vi "UHR-Fleezers Control (fpga) - 11.4c.vi"() -> ()   [LabVIEW 2012]
doc: "UHR-Fleezers Instrument Control Code (fpga)"
uses:
  <vilib>/Platform/TimedLoop/XDataNode/timing_clust.ctl
  <vilib>/Platform/TimedLoop/XDataNode/nitl_modes.ctl
  <vilib>/Platform/TimedLoop/XDataNode/wakeup.ctl
  <vilib>/rvi/eio/common/nirviEmuTemplateMethod_errors.vi
  <vilib>/rvi/Emulation/niFpgaSctlEmulationGetInTimedLoop.vi
  <vilib>/rvi/DataTransferAndStorage/Container/Common/niFpgaContainerGetUniqueNameForEmu.vi
  <vilib>/rvi/FIFO/Fifo_Resource/nirvififoEmulationSetSize.vi
  <vilib>/rvi/Emulation/niFpgaSctlEmulationFifoFullMgr.vi
  <vilib>/rvi/errors/niFpgaSetErrorForExecOnDevCompSimple.vi
  <vilib>/rvi/eio/common/nirviEmuReportErrorAndStop.vi
  <vilib>/rvi/interface/RandomDataEmulation/nirviRandomDataFPGAFIFO.vi
  <vilib>/rvi/interface/RandomDataEmulation/niFpgaRandomDataHandleErrors.vi
  <vilib>/rvi/Emulation/niFpgaSctlEmulationGlobalWrite.vi
  <vilib>/rvi/Emulation/niFpgaSctlEmulationRegisterWithScheduler.vi
  <vilib>/rvi/Emulation/niFpgaSctlEmulationScheduler.vi
  <vilib>/rvi/Emulation/niFpgaSctlEmulationResourceMgr.vi
  <vilib>/Platform/TimedLoop/XDataNode/XDataNode.xnode
  <vilib>/eio/EIOMethodNode/EIOMethodNode.xnode
  <vilib>/eio/EIONode/EIONode.xnode
  <vilib>/rvi/DataTransferAndStorage/Container/XNode/niFpgaContainer.xnode
  <vilib>/rvi/FIFO/Fifo_Resource/nirvififoEmulationRead.vi
  <vilib>/rvi/interface/RandomDataEmulation/nirviRandomDataFpgaReadWriteTemplate.vi
  <vilib>/rvi/FIFO/Fifo_Resource/nirvififoEmulationWrite.vi
  <vilib>/addons/control/pid/fpga.llb/XNode/niFpgaPID.xnode
  <vilib>/Platform/TimedLoop/XDataNode/XDNodeRunTimeDep.lvlib
panel:
  in  "Tab Control":T1(tab)=enum."Force FB"
  in  "Set 3":bool
  in  "Set 2":bool=TRUE
  in  "Set 1":bool=TRUE
  in  "Trap Pos to FIFO":bool
  in  "N of AI1 Int Acq Sets":i16=2 min=1 max=3 step=1
  out "AI Late Counter":u8
  in  "ai count":u16=400
  in  "+ phase":bool
  in  "Phase count adjustment":i16
  out "Relative phase":i16
  in  "AI to FIFO":bool
  out "BD1 Frequency Out 1":u64
  out "BD1 Frequency Out 2":u64
  out "Trap Pos FIFO Timeout":u16
  out "Trap AI FIFO Timeout":u16
  in  "Trap FIFO Set Timeout":i32
  in  "Tab Control 2":T2(tab)
  in  "RD":bool
  in  "FB1 output high":i16=3000
  in  "FB1 output low":i16
  in  "D1":i16
  in  "I1":i16=5
  in  "P1":i16=10
  in  "Swap F1 and F2":bool
  in  "Cont. Scan":bool
  in  "Abort scan":bool
  in  "Cycles per step":u64
  in  "Scan BD":bool
  in  "Number of scans":u16
  in  "Scan steps":u64
  in  "Scan freq.  increment":i64
  out "Scanning":bool
  in  "Start scan":bool
  in  "OSK Bd 1":bool
  in  "Reset Bd 1":bool
  in  "PMODE":bool
  in  "Direct RF Box \nCommunication":bool
  in  "Data BD 2":u8 format="%08b"
  in  "Data BD 1":u8 format="%08b"
  in  "Address":u8 format="%02x"
  in  "Update Data":bool
  in  "FPGA Controls\n RF Box":bool
  in  "Number Interlace Cycles":u8=2 min=1 max=3
  in  "Interlace Off Parameters":u8=1 min=1 max=3
  in  "Interlace ON/OFF":bool
  out "DIO Relative phase":i16
  in  "Phase count adjustment (DIO)":i16
  in  "+ phase (DIO)":bool
  out "DIO Late Counter":u8
  in  "DIO count 1 (ticks)":u16=400
  in  "DIO count 2 (ticks)":u16=400
  in  "DIO count 3 (ticks)":u16=400
  out "AI2 Y Sum Set 2":i16
  out "AI2 Y Sum Set 1":i16
  in  "FB Setpoint Set 1":i16 min=0 step=1
  in  "FB Reset Set 1":bool
  in  "FB On/Off Set 1":bool
  in  "FB Reset Set 2":bool
  in  "FB On/Off Set 2":bool
  in  "FB Setpoint Set 2":i16 min=0 step=1
  out "Scan I":u64
  in  "Amp switch delay":u8=5
  in  "XY phase ext loop method":bool
  in  "BD 2 Amplitude 1":u16
  in  "BD 1 Amplitude 1":u16
  in  "BD 2 Frequency 1":u64
  in  "BD 1 Frequency 1":u64
  in  "BD 2 Amplitude 2":u16
  in  "BD 1 Amplitude 2":u16
  in  "BD 2 Frequency 2":u64
  in  "BD 1 Frequency 2":u64
  in  "BD 2 Amplitude 3":u16
  in  "BD 1 Amplitude 3":u16
  in  "BD 2 Frequency 3":u64
  in  "BD 1 Frequency 3":u64
  in  "BD 1 Delay (ticks)":u8
  in  "BD 2 Delay (Ticks)":u8 caption="Count(Ticks)"
  in  "Next trap write delay (ticks)":u8 caption="Count(Ticks)"
  in  "Amp switch delay 2":u8=5
  in  "BD 2 Delay (Ticks) 2":u8 caption="Count(Ticks)"
  in  "BD 1 Delay (ticks) 2":u8
  in  "FB2 output high":fxp<+/-,16,1>=0.999969482421875
  in  "FB2 output low":fxp<+/-,16,1>=-1.0
  in  "P2":fxp<+/-,16,8> format="%.11g"
  in  "I2":fxp<+/-,16,8>=10.0 format="%.11g"
  in  "D2":fxp<+/-,16,8> format="%.11g"
  in  "Negate Diff?":bool
  in  "Diff FB Measurement?":bool
  in  "FB Trig Integrate":u32=1
  out "TTrig?":bool
  in  "TTrig Negate Pos":bool=TRUE
  out "Trap Pos FB Int Signal":fxp<+/-,24,9> format="%.18g"
  out "Trap Pos FB Int-Norm Signal":fxp<+/-,16,1> format="%.16g"
  in  "FPGA TTrig Thresh":i64
  in  "FPGA Trap Trig":bool
  out "Trap Pos FB Action":i64
  in  "Trap Pos. FB Offset Factor":i64
  in  "Trap Pos. FB Mult Factor":i64=2
  in  "Trap Pos. FB Reset":bool
  in  "Trap Pos FB Monitor T1 or T2":bool
  in  "AI1 X Scale":u16
  in  "Trap Pos FB Int Count":u16=100
  in  "Trap Pos FB Negate Action":bool
  out "AI1 X Set 2":fxp<+/-,16,1>
  out "AI1 X Set 1":fxp<+/-,16,1>
  in  "Trap Pos. FB SP":fxp<+/-,16,1>
  in  "Force feedback":bool
  out "TTrig Sig":i64
  out "TTrig Fin Thresh":i64
  in  "1D or 2D Scan?":bool
  in  "Abort scan (MCL)":bool
  in  "MCL Scan Axis":bool
  in  "Cont. Scan (MCL)":bool
  out "Scan I (MCL)":u64
  in  "Number of scans (MCL)":u16
  out "Scanning MCL":bool
  in  "Scan steps (MCL)":u64
  in  "Cycles per step (MCL)":u64
  in  "Scan freq.  increment (MCL)":i16
  in  "Start scan (MCL)":bool
  in  "AO2":i16
  in  "AO1":i16
  out "MCL Late Counter":u8
  in  "MCL count":u32=800
  out "MCL Relative Phase":i16
  in  "Phase count adjustment (MCL)":i16
  in  "+ phase (MCL)":bool
  out "APD3 out state":bool
  in  "APD Gate Operating Mode":u8 max=2 step=1
  in  "Invert APD Gate":bool
  in  "APD Gate OFF Count":u16=100
  in  "APD Gate ON Count":u16=300
  out "APD 1 Gate Late Counter":u8
  out "APD 1 Gate Relative Phase":i16
  in  "Phase count adjustment (APD 1 Gate)":i16
  in  "+ phase (APD 1 Gate)":bool
  out "APD 2 Counts 0":u32
  out "APD 2 Counts 1":u32
  out "APD 1 Counts 0":u32
  out "APD 1 Counts 1":u32
  out "APD1 out state":bool
  in  "APD AO scale factor":i16=1
  in  "APD to FIFO":bool
  in  "APD Acq Rate Count":u32=20000000
  out "APD Acq Late Counter":u8
  out "APD Acq Relative Phase":i16
  in  "Phase Count Adjustment (APD Acq)":i16
  in  "+ phase (APD Acq)":bool
  in  "Phase count adjustment (APD 2 Gate)":i16
  out "APD 2 Gate Late Counter":u8
  out "APD 2 Gate Relative Phase":i16
  in  "+ phase (APD 2 Gate)":bool
  out "APD2 out state":bool
  out "APD 3 Counts 0":u32
  out "APD 3 Counts 1":u32
  out "APD 3 Gate Late Counter":u8
  in  "Phase count adjustment (APD 3 Gate)":i16
  out "APD 3 Gate Relative Phase":i16
  in  "+ phase (APD 3 Gate)":bool
  in  "D3":i16
  in  "I3":i16=5
  in  "P3":i16=10
  in  "Green Filter Flipper":bool
  in  "Green FB Count":u16=1200
  out "Green Late Counter":u8
  out "Green FB Relative Phase":i16
  in  "Phase count adjustment (Green FB)":i16=10
  in  "+ phase (Green FB)":bool
  out "Green FB Sum":i16
  in  "Green int current ON count adj":u16=150
  in  "Current Out":u16=30000
  in  "Green FB On/Off":bool
  in  "Green FB Setpoint":i16=250 min=0 step=1
  in  "Green FB Reset":bool
  in  "Operating Mode 2":u8=2 max=2 step=1
  in  "Invert GI 2":bool
  in  "Green interlace OFF count 2":u16=900
  in  "Green interlace ON count 2":u16=300
  out "GI Late Counter 2":u8
  out "GI Relative phase 2":i16
  in  "Phase count adjustment (GI) 2":i16=20
  in  "+ phase (GI) 2":bool
  in  "Green interlace OFF count":u16=100
  out "GI Relative phase":i16
  in  "Phase count adjustment (GI)":i16
  in  "+ phase (GI)":bool
  in  "Green interlace ON count":u16=300
  out "GI Late Counter":u8
  in  "Invert GI":bool
  in  "Operating Mode":u8 max=2 step=1
  in  "+ phase (RI)":bool
  out "RI Relative phase":i16
  out "RI Late Counter":u8
  in  "Red interlace ON count":u16=300
  in  "Red interlace OFF count":u16=100
  in  "Invert RI":bool
  in  "Red Laser Operating Mode":u8 max=2 step=1
  in  "Phase count adjustment (RI)":i16
  out "Red FB Intensity":i16
  in  "RI Current Out":u16=30000
  in  "Red FB On/Off":bool
  in  "D4":i16
  in  "I4":i16=5
  in  "P4":i16=10
  in  "Red FB Setpoint":i16=250 min=0 step=1
  in  "Red FB Reset":bool
  in  "RI Operating Mode 2":u8=2 max=2 step=1
  in  "Invert RI 2":bool
  in  "Phase count adjustment (BI AO)":i16=20
  in  "Blue current ON count adj (AO)":u16=150
  in  "BI Current Out":i16=30000
  in  "Blue FB On/Off":bool
  in  "D5":i16
  in  "I5":i16=5
  in  "P5":i16=10
  in  "Blue FB Setpoint":i16=250 min=0 step=1
  in  "Blue FB Reset":bool
  in  "BI Operating Mode (AO)":u8=2 max=2 step=1
  in  "Invert BI (AO)":bool
  in  "Blue OFF count (AO)":u16=900
  in  "Blue ON count (AO)":u16=300
  out "BI Late Counter (AO)":u8
  out "BI Relative phase (AO)":i16
  in  "+ phase (BI AO)":bool
  in  "Phase count adjustment (BI D)":i16
  in  "Blue Laser Operating Mode (D)":u8 max=2 step=1
  in  "Invert BI (D)":bool
  in  "Blue interlace OFF count (D)":u16=100
  in  "Blue interlace ON count (D)":u16=300
  out "Blue Late Counter (D)":u8
  out "BI Relative phase (D)":i16
  in  "+ phase (BI D)":bool
  out "Blue Intensity":i16
  # "Only one of these can be on\nat a time:"
  # "Raster Scan AOD"
  # "1 (X)"
  # "2 (Y)"
  # "IR Intensity Feedback (RF BD 1)"
  # "FB Gains Set 1"
  # "FB output range 1"
  # "False is usual, True is external loop method"
  # "Parameters if using the external RF switching loop"
  # "Parameters if using the usual internal RF switching method"
  # "FB Triggering Excitation Laser"
  # "Trap Pos. FB Gains"
  # "Trap Pos. FB Range"
  # "AO1 (Y)"
  # "2D"
  # "1D"
  # "AO2 (X)"
  # "APD AO for aligning"
  # "Detection Loop"
  # "Green fluorescent laser digital gate interlacing loop"
  # "0 Forced ON\n1 Forced OFF\n2 Interlacing"
  # "Green FB Gains"
  # "Red fluorescent laser digital gate interlacing loop"
  # "Detection Loop"
  # "0 Forced ON\n1 Forced OFF\n2 Interlacing"
  # "Analog/FB Control Loop\n(Disabled)"
  # "Digital Control Loop"
  # "Blue laser intensity reading"
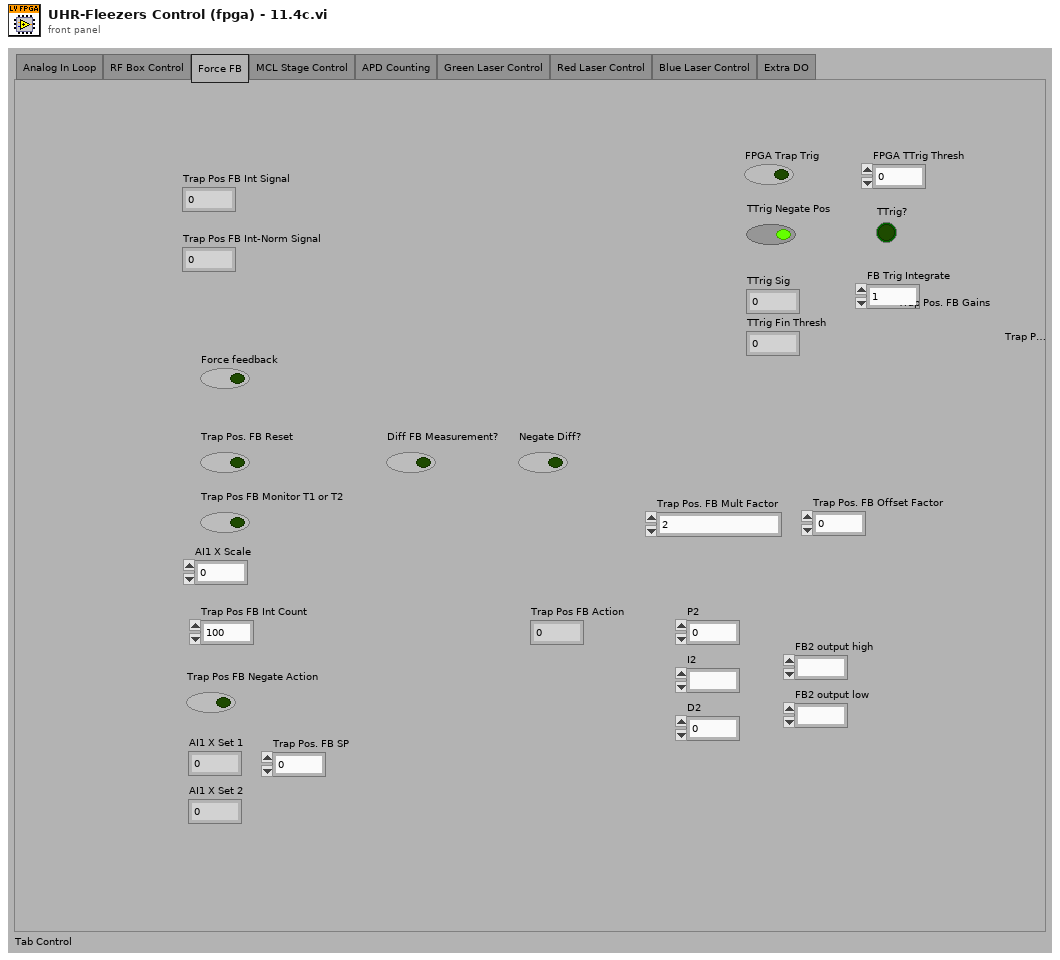
[diagram p1: front panel]
types:
  T1 = enum32{"Analog In Loop", "RF Box Control", "Force FB", "MCL Stage Control", "APD Counting", "Green Laser Control", "Red Laser Control", "Blue Laser Control", "Extra DO"}
  T2 = enum32{"Controls", "Interlacing Frequency and Amplitude Values"}
  T3 = typedef "XDNodeRunTimeDep.lvlib/timing_clust.ctl" = cluster{"Expected End [f-1]":u64, "Actual End [f-1]":u64, "Finished Late? [f-1]":bool, "Expected End [i-1]":u64, "Actual End [i-1]":u64, "Finished Late? [i-1]":bool, "Expected Start [i]":u64, "Actual Start [i]":u64, "Expected Start [f]":u64, "Actual Start [f]":u64, "Source Name":string, "Structure Name":string, "Period":i64, "Deadline":i64, "Offset":i64, "Start":i64, "Priority":i32, "Timeout":i32, "Mode":T4, "Wakeup Reason":T5, "Error":errorcluster, "Source Type":string, "Secondary Source Type":string, "Global End Time":u64, "Global Start Time":u64, "Frame Duration":u64, "Iteration Duration":u64, "Assigned CPU":i32, "I/O Scan Engine Mode":u32}
  T4 = typedef "XDNodeRunTimeDep.lvlib/nitl_modes.ctl" = enum32{"No Change", "Process missed periods, maintain original phase", "Discard missed periods, maintain original phase", "Process missed periods, ignore original phase", "Discard missed periods, ignore original phase"}
  T5 = typedef "XDNodeRunTimeDep.lvlib/wakeup.ctl" = enum32{"Normal", "Aborted", "Asynchronous wakeup", "Timing source error", "Timed loop error", "Timeout"}
  T6 = cluster{"proportional gain (Kc)":i16, "integral gain (Kc*Ts/Ti)":i16, "derivative gain (Kc*Td/Ts)":i16}
  T7 = cluster{"FB1 output high":i16, "FB1 output low":i16}
  T8 = cluster{"P2":fxp<+/-,16,8>, "I2":fxp<+/-,16,8>, "D2":fxp<+/-,16,8>}
  T9 = cluster{"FB2 output high":fxp<+/-,16,1>, "FB2 output low":fxp<+/-,16,1>}
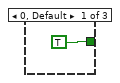
[diagram p3: hidden frame]
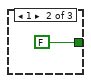
[diagram p4: hidden frame]
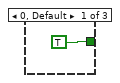
[diagram p5: hidden frame]
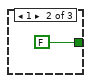
[diagram p6: hidden frame]
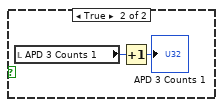
[diagram p7: hidden frame]
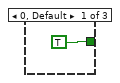
[diagram p8: hidden frame]
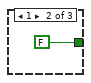
[diagram p9: hidden frame]
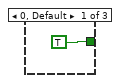
[diagram p10: hidden frame]
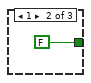
[diagram p11: hidden frame]
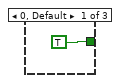
[diagram p12: hidden frame]
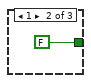
[diagram p13: hidden frame]
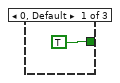
[diagram p14: hidden frame]
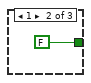
[diagram p15: hidden frame]
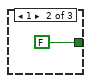
[diagram p18: hidden frame]
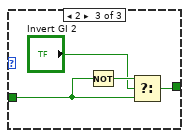
[diagram p19: hidden frame]
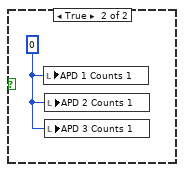
[diagram p20: hidden frame]
diagram:
  w3 = u16 0
  w5 = FALSE
  w2 = FALSE
  # "timing array current index"
  # "timing array"
  # "timing counter (phase adjusted here)"
  # "late counter"
  n1 = while "External XY RF switching timing loop" {
    stop <- FALSE stop-if-true
    # "This loop is stalled until the RF FIFO get a value, which only happens if we are using the external loop RF switching method. With this method we gain additional delay time (because \nwe allow the rest of the main RF loop to procede while this loop waits to send the switch signals - a form of parallelism). Probably this is always the method to use. Helps to simplify \nthe main RF code. If it works reliably, could take out the redundant code in the main RF loop to save space and simplify."
    n2 = xnode "FIFO Read"("Timeout"=-1) -> ("Element"=w15:bool)  [unwired: 1 in, 2 out]
    n3 = flat-sequence "BD 1 (X)" {
      tunnel: w15 -> [w24]
      tunnel: [w24] -> w14
      tunnel: w14 -> [w26]
      tunnel: "Amp switch delay 2" -> [w27]
      frame #0 {
        n4 = call "Wait9"("Count(Ticks)"="BD 1 Delay (ticks) 2") -> ()  [unwired: 1 out]
      }
      frame #1 {
        # "switch frequency"
        n5 = xnode "FPGA I/O Node"("Connector1/DIO36"=w26) -> ()  [unwired: 1 in, 1 out]
      }
      frame #2 {
        # "~5 ticks is usual"
        n6 = call "Wait10"("Count(Ticks)"=w27) -> ()  [unwired: 1 out]
      }
      frame #3 {
        # "this switches amplitude"
        # "switch amplitude"
        # "send udclk high"
        n7 = xnode "FPGA I/O Node"("Connector1/DIO30"=TRUE ("Connector1/DIO15")) -> ()  [unwired: 1 in, 1 out]
      }
      frame #4 {
        # "reset to be ready for next\ncycle"
        # "send udclk low"
        n8 = xnode "FPGA I/O Node"("Connector1/DIO30"=FALSE ("Connector1/DIO15")) -> ()  [unwired: 1 in, 1 out]
      }
    }
    n9 = flat-sequence "BD 2 (Y)" {
      tunnel: w15 -> [w18]
      tunnel: [w18] -> w13
      tunnel: w13 -> [w20]
      tunnel: "Amp switch delay 2" -> [w21]
      frame #0 {
        n10 = call "Wait11"("Count(Ticks)"="BD 2 Delay (Ticks) 2") -> ()  [unwired: 1 out]
      }
      frame #1 {
        # "switch frequency"
        n11 = xnode "FPGA I/O Node"("Connector1/DIO37"=w20) -> ()  [unwired: 1 in, 1 out]
      }
      frame #2 {
        # "~5 ticks is usual"
        n12 = call "Wait12"("Count(Ticks)"=w21) -> ()  [unwired: 1 out]
      }
      frame #3 {
        # "this switches amplitude"
        # "switch amplitude"
        # "send udclk high"
        n13 = xnode "FPGA I/O Node"("Connector1/DIO29"=TRUE ("Connector1/DIO15")) -> ()  [unwired: 1 in, 1 out]
      }
      frame #4 {
        # "reset to be ready for next\ncycle"
        # "send udclk low"
        n14 = xnode "FPGA I/O Node"("Connector1/DIO29"=FALSE ("Connector1/DIO15")) -> ()  [unwired: 1 in, 1 out]
      }
    }
  }
  n15 = flat-sequence "FPGA initialization to do before running any of the loops" {
    tunnel: [u16 0 ("DIO count 3 (ticks)")] -> w1
    tunnel: [w31] -> _
    frame #0 {
      w30 = FALSE ("Enable")
      # "BD 2 (Y)"
      # "BD 1 (X)"
      # "Start up expansion chassis early\nto avoid delays later"
      # "This pin controls udclk on the RF boards.\nWhen initially configuring the boards, this pin needs to be\nconfigured as a high impedance input.  Later it will be switched\nto an output."
      # "Initial setting of DIO data and \naddress to low (before reset).  \nThis needs to happen before the other\ncontrol method loops execute."
      n16 = xnode "FPGA I/O Node"("Chassis2/Mod4/AO0"=u16 0) -> ("Chassis2/Mod1/AI0"=w31:i16)  [unwired: 2 in, 2 out]
      n17 = xnode "FPGA I/O Method Node"("Enable"=w30) -> ()  [unwired: 1 in, 1 out]
      n18 = xnode "FPGA I/O Method Node"("Enable"=w30) -> ()  [unwired: 1 in, 1 out]
      n19 = xnode "FPGA I/O Node"("Connector1/DIO0"=FALSE, "Connector1/DIO1"=FALSE, "Connector1/DIO2"=FALSE, "Connector1/DIO3"=FALSE, "Connector1/DIO4"=FALSE, "Connector1/DIO5"=FALSE, "Connector1/DIO6"=FALSE, "Connector1/DIO7"=FALSE, "Connector1/DIO8"=FALSE, "Connector1/DIO9"=FALSE, "Connector1/DIO10"=FALSE, "Connector1/DIO11"=FALSE, "Connector1/DIO12"=FALSE, "Connector1/DIO13"=FALSE, "Connector1/DIO15"=FALSE, "Connector1/DIO20"=FALSE, "Connector1/DIO21"=FALSE, "Connector1/DIO22"=FALSE, "Connector1/DIO23"=FALSE, "Connector1/DIO24"=FALSE, "Connector1/DIO25"=FALSE, "Connector1/DIO26"=FALSE, "Connector1/DIO27"=FALSE, "Connector1/DIO14"=FALSE) -> ()  [unwired: 24 in, 24 out]
    }
  }
  n20 = local read "AO1"() -> (w10:i16)
  n21 = local read "AO2"() -> (w9:i16)
  n22 = node-c288() -> (w8:T3)  [unwired: 1 in]
  n23 = timed-loop "RF box board DIO control: control bits" {
    timing: w8 -> [_]
    timing-out: [_] -> w7
    tunnel: [w60] -> _
    tunnel: w1 -> [w60]
    stop <- FALSE stop-if-true
    n24 = xnode "FPGA I/O Node"("Connector1/DIO16"="RD", "Connector1/DIO17"="PMODE", "Connector1/DIO18"="OSK Bd 1", "Connector1/DIO19"="Reset Bd 1", "Connector0/DIO3"="Green Filter Flipper") -> ()  [unwired: 5 in, 5 out]
  }
  n25 = while "RF box board DIO control: parallel communication" {
    shift-right: [w73] -> _
    shift-left: w1 -> [w72]
    shift-right: [w71] -> _
    shift-left: FALSE ("Swap F1 and F2") -> [w70]
    stop <- FALSE stop-if-true
    n26 = flat-sequence {
      tunnel: w70 -> [w77]
      tunnel: w72 -> [w75]
      tunnel: [w77] -> w69
      tunnel: [w76] -> w68
      tunnel: [w75] -> w67
      tunnel: [w83] -> w73
      tunnel: [w82] -> w71
      tunnel: w69 -> [w81]
      tunnel: w68 -> [w79]
      tunnel: w67 -> [w78]
      frame #0 {
        n27 = call "Loop Timer"("Count(Ticks)"=w75) -> ("Tick Count(Ticks)"=w76:u16)
      }
      frame #1 {
        n28 = flat-sequence {
          tunnel: ["FPGA Controls\n RF Box"] -> w80
          tunnel: w81 -> [w84]
          tunnel: [w138] -> w83
          tunnel: [w151] -> w82
          tunnel: w80 -> [w150]
          tunnel: w79 -> [w144]
          tunnel: w78 -> [w141]
          frame #0 {
            n29 = case shown="True" "FPGA Controls\n RF Box" {
              tunnel: w84 -> [_ w86]
              frame False {
              }
              frame True {
                n30 = flat-sequence {
                  tunnel: w86 -> [w96]
                  frame #0 {
                    n31 = First Call?() -> (First Call?: T/F=w87:bool)
                    n32 = case shown="True" w87 {
                      frame False {
                      }
                      frame True {
                        # "BD 2"
                        # "BD 1"
                        # "If first time data updated, be sure to set WR high and UDCLK low\nbefore setting data and address bits."
                        n33 = xnode "FPGA I/O Method Node"("Enable"=TRUE) -> ("FPGA I/O Out"=w89:refnum<k21>)  [unwired: 1 in]
                        n34 = xnode "FPGA I/O Method Node"("Enable"=TRUE) -> ("FPGA I/O Out"=w92:refnum<k21>)  [unwired: 1 in]
                        n35 = xnode "FPGA I/O Node"("Connector1/DIO15"=TRUE) -> ()  [unwired: 1 in, 1 out]
                        n36 = xnode "FPGA I/O Node"("I/O Item"=FALSE ("Connector1/DIO30"), "FPGA I/O In"=w89) -> ()  [unwired: 1 out]
                        n37 = xnode "FPGA I/O Node"("I/O Item"=FALSE ("Connector1/DIO30"), "FPGA I/O In"=w92) -> ()  [unwired: 1 out]
                      }
                    }
                  }
                  frame #1 {
                    n38 = case shown="True" "XY phase ext loop method" {
                      tunnel: w96 -> [w98 w110]
                      frame False {
                        # "Usual operation"
                        n39 = flat-sequence "BD 1 (X)" {
                          tunnel: w98 -> [w105]
                          tunnel: "Amp switch delay" -> [w106]
                          frame #0 {
                            n40 = call "Wait6"("Count(Ticks)"="BD 1 Delay (ticks)") -> ()  [unwired: 1 out]
                          }
                          frame #1 {
                            # "switch frequency"
                            n41 = xnode "FPGA I/O Node"("Connector1/DIO36"=w105) -> ()  [unwired: 1 in, 1 out]
                          }
                          frame #2 {
                            # "~5 ticks is usual"
                            n42 = call "Wait4"("Count(Ticks)"=w106) -> ()  [unwired: 1 out]
                          }
                          frame #3 {
                            # "this switches amplitude"
                            # "switch amplitude"
                            # "send udclk high"
                            n43 = xnode "FPGA I/O Node"("Connector1/DIO30"=TRUE ("Connector1/DIO15")) -> ()  [unwired: 1 in, 1 out]
                          }
                          frame #4 {
                            # "reset to be ready for next\ncycle"
                            # "send udclk low"
                            n44 = xnode "FPGA I/O Node"("Connector1/DIO30"=FALSE ("Connector1/DIO15")) -> ()  [unwired: 1 in, 1 out]
                          }
                        }
                        n45 = flat-sequence "BD 2 (Y)" {
                          tunnel: w98 -> [w100]
                          tunnel: "Amp switch delay" -> [w101]
                          frame #0 {
                            n46 = call "Wait7"("Count(Ticks)"="BD 2 Delay (Ticks)") -> ()  [unwired: 1 out]
                          }
                          frame #1 {
                            # "switch frequency"
                            n47 = xnode "FPGA I/O Node"("Connector1/DIO37"=w100) -> ()  [unwired: 1 in, 1 out]
                          }
                          frame #2 {
                            # "~5 ticks is usual"
                            n48 = call "Wait5"("Count(Ticks)"=w101) -> ()  [unwired: 1 out]
                          }
                          frame #3 {
                            # "this switches amplitude"
                            # "switch amplitude"
                            # "send udclk high"
                            n49 = xnode "FPGA I/O Node"("Connector1/DIO29"=TRUE ("Connector1/DIO15")) -> ()  [unwired: 1 in, 1 out]
                          }
                          frame #4 {
                            # "reset to be ready for next\ncycle"
                            # "send udclk low"
                            n50 = xnode "FPGA I/O Node"("Connector1/DIO29"=FALSE ("Connector1/DIO15")) -> ()  [unwired: 1 in, 1 out]
                          }
                        }
                      }
                      frame True {
                        # "Operation when you need a long delay for either X or Y to synchonize AOD light out phase (> ~100 ticks)."
                        # "Trigger the external loop by sending the boolean FSK value through a FIFO"
                        n51 = xnode "FIFO Write"("Element"=w110, "Timeout"=-1) -> ()  [unwired: 1 in, 2 out]
                      }
                    }
                  }
                }
              }
            }
          }
          frame #1 {
            # "This is the prior cycle's on time"
            # "increment timing\nindex, reset to 0 if \nend of matrix"
            # "Reset to begginning (1) when number of cycles reached."
            # "timing index"
            # "build byte stacks for writing data\n(must correspond to addresses array constant)"
            # "Timing housekeeping"
            # "Adjust phase if late\n(maintains constant phase relationship between cycles)"
            n52 = Bundle("FB1 output high"="FB1 output high", "FB1 output low"="FB1 output low") -> (w111:T7)  [unwired: 1 in]
            n53 = Bundle("P1"="P1", "I1"="I1", "D1"="D1") -> (w112:cluster{"P1":i16, "I1":i16, "D1":i16})  [unwired: 1 in]
            n54 = feedback #1(u8 0 ("t")) -> (w147:u8)
            n55 = Increment(x=w147) -> (x+1=w191:u8)
            n56 = Increment(x="Number Interlace Cycles") -> (x+1=w186:u8)
            n57 = Equal?(x=w191, y=w186) -> (x = y?=w193:bool)
            n58 = Select(t=u8 1, s=w193, f=w191) -> (s? t:f=w146:u8)
            n59 = feedback-in #1(w146) -> ()
            n60 = Increment(x=w146) -> (x+1=w188:u8)
            n61 = Equal?(x=w188, y=w186) -> (x = y?=w189:bool)
            n62 = Select(t=u8 1, s=w189, f=w188) -> (s? t:f=w185:u8)
            n63 = Select(t=w185, s="Interlace ON/OFF", f="Interlace Off Parameters") -> (s? t:f=w169:u8)
            n64 = case shown="1, Default" w169 {
              tunnel: [w270 "BD 1 Frequency 2" "BD 1 Frequency 3"] -> w181
              tunnel: [w269 "BD 2 Frequency 2" "BD 2 Frequency 3"] -> w170
              tunnel: ["BD 2 Amplitude 1" "BD 2 Amplitude 2" "BD 2 Amplitude 3"] -> w126
              tunnel: [w258 w429 "BD 1 Amplitude 3"] -> w129
              tunnel: w112 -> [w232 w426 _]
              tunnel: w111 -> [w233 w425 _]
              frame 1, Default {
                w249 = fxp<+/-,24,9> 0.0 ("AI1 X Set 2")
                w242 = u16 0
                w265 = u64 0 ("f")
                # "This signal integration happens no matter what\nso that correct setpoints can be chosen before \nturning on the FB."
                # "Trap 1"
                n65 = local read "AI1 X Set 2"() -> (w245:fxp<+/-,16,1>)
                n66 = local read "AI1 X Set 1"() -> (w246:fxp<+/-,16,1>)
                n67 = local read "Scanning"() -> (w271:bool)
                n68 = Or(x=w271, y="Start scan") -> (x .or. y?=w263:bool)
                n69 = case shown="False" "Diff FB Measurement?" {
                  tunnel: w245 -> [w279 w288]
                  tunnel: w246 -> [w278 w289]
                  tunnel: [w276 w280] -> w247
                  frame False {
                    n70 = Select(t=w278, s="Trap Pos FB Monitor T1 or T2", f=w279) -> (s? t:f=w276:fxp<+/-,16,1>)
                  }
                  frame True {
                    n71 = Subtract(x=w289, y=w288) -> (x-y=w281:fxp<+/-,17,2>)
                    n72 = Not(x="Negate Diff?") -> (.not. x?=w287:bool)
                    n73 = Boolean To (0,1)(Boolean="Negate Diff?") -> (0, 1=w285:i16)
                    n74 = Boolean To (0,1)(Boolean=w287) -> (0, 1=w286:i16)
                    n75 = Negate(x=w285) -> (-x=w284:i16)
                    n76 = Add(x=w284, y=w286) -> (x+y=w282:i16)
                    n77 = Multiply(x=w282, y=w281) -> (x*y=w280:fxp<+/-,32,17>)
                  }
                }
                n78 = Not(x="Abort scan") -> (.not. x?=w261:bool)
                n79 = And(x=w261, y=w263) -> (x .and. y?=w260:bool)
                n80 = case "For raster scanning" shown="True" w260 {
                  tunnel: [u64 0 w415] -> w266
                  tunnel: "Start scan" -> [_ w400]
                  frame False {
                    n81 = local write "Scanning"(FALSE ("scanning")) -> ()
                  }
                  frame True {
                    w384 = i64 0
                    w383 = u64 0
                    # "scan incr."
                    # "freq. incr. mult."
                    # "count steps"
                    # "count number of cycles"
                    n82 = feedback #2(w383) -> (w412:u64)
                    n83 = Select(t=w383, s=w400, f=w412) -> (s? t:f=w414:u64)
                    n84 = Increment(x=w414) -> (x+1=w411:u64)
                    n85 = Greater?(x="Cycles per step", y=w411) -> (0:w393:bool)
                    n86 = Select(t=w411, s=w393, f=w383) -> (s? t:f=w410:u64)
                    n87 = feedback-in #2(w410) -> ()
                    n88 = feedback #3(w383) -> (w409:u64)
                    n89 = Select(t=w383, s=w400, f=w409) -> (s? t:f=w404:u64)
                    n90 = Increment(x=w404) -> (x+1=w408:u64)
                    n91 = Add(x="Scan steps", y="Scan steps") -> (x+y=w407:u64)
                    n92 = Select(t=w404, s=w393, f=w408) -> (s? t:f=w388:u64)
                    n93 = Greater?(x=w407, y=w388) -> (0:w387:bool)
                    n94 = Select(t=w388, s=w387, f=w383) -> (s? t:f=w405:u64)
                    n95 = feedback-in #3(w405) -> ()
                    n96 = Equal?(x="Scan steps", y=w388) -> (x = y?=w392:bool)
                    n97 = Greater?(x="Scan steps", y=w404) -> (0:w403:bool)
                    n98 = feedback #4(w384) -> (w406:i64)
                    n99 = Select(t=w384, s=w400, f=w406) -> (s? t:f=w390:i64)
                    n100 = Increment(x=w390) -> (x+1=w402:i64)
                    n101 = Decrement(x=w390) -> (x-1=w401:i64)
                    n102 = Select(t=w402, s=w403, f=w401) -> (s? t:f=w391:i64)
                    n103 = Select(t=w390, s=w392, f=w391) -> (s? t:f=w389:i64)
                    n104 = Select(t=w390, s=w393, f=w389) -> (s? t:f=w385:i64)
                    n105 = Select(t=w385, s=w387, f=w384) -> (s? t:f=w386:i64)
                    n106 = feedback-in #4(w386) -> ()
                    n107 = feedback #5(w383) -> (w399:u64)
                    n108 = Select(t=w383, s=w400, f=w399) -> (s? t:f=w395:u64)
                    n109 = Increment(x=w395) -> (x+1=w396:u64)
                    n110 = Select(t=w395, s=w387, f=w396) -> (s? t:f=w394:u64)
                    n111 = Greater?(x="Number of scans", y=w394) -> (0:w380:bool)
                    n112 = Multiply(x="Scan freq.  increment", y=w390) -> (x*y=w415:i64)
                    n113 = Select(t=TRUE, s="Cont. Scan", f=w380) -> (s? t:f=w379:bool)
                    "Scanning" <- w379
                    n114 = Select(t=w394, s=w379, f=w383) -> (s? t:f=w397:u64)
                    n115 = feedback-in #5(w397) -> ()
                    n116 = Increment(x=w394) -> (x+1=→"Scan I":u64)
                  }
                }
                n117 = feedback #6(w242) -> (w241:u16)
                n118 = Increment(x=w241) -> (x+1=w243:u16)
                n119 = Greater Or Equal?(x=w243, y="Trap Pos FB Int Count") -> (x >= y?=w234:bool)
                n120 = Select(t=w242, s=w234, f=w243) -> (s? t:f=w244:u16)
                n121 = feedback-in #6(w244) -> ()
                n122 = feedback #7(w249) -> (w248:fxp<+/-,24,9>)
                n123 = Add(x=w247, y=w248) -> (x+y=w240:fxp<+/-,24,9>)
                n124 = case "For intensity feedback" shown="True" "FB On/Off Set 1" {
                  tunnel: "BD 1 Amplitude 1" -> [w417 _]
                  tunnel: [w417 w421] -> w258
                  tunnel: w233 -> [_ w418]
                  tunnel: w232 -> [_ w419]
                  frame False {
                  }
                  frame True {
                    n125 = local read "AI2 Y Sum Set 1"() -> (w422:i16)
                    n126 = call "Slower PID.vi"("process variable"=w422, "reset?"="FB Reset Set 1", "setpoint"="FB Setpoint Set 1", "PID gains (x 2^8)"=w419, "output range"=w418) -> ("output"=w423:i16)  [unwired: 10 out]
                    n127 = To Unsigned Word Integer(number=w423) -> (unsigned 16bit integer=w421:u16)
                  }
                }
                n128 = Select(t=w249, s=w234, f=w240) -> (s? t:f=w252:fxp<+/-,24,9>)
                n129 = feedback-in #7(w252) -> ()
                n130 = Divide(x=w240, y="Trap Pos FB Int Count") -> (x/y=w235:fxp<+/-,16,1>)
                n131 = feedback #8(fxp<+/-,24,9> 0.0 ("AI1 X Set 2")) -> (w253:fxp<+/-,24,9>)
                n132 = Select(t=w240, s=w234, f=w253) -> (s? t:f=w254:fxp<+/-,24,9>)
                "Trap Pos FB Int Signal" <- w254
                n133 = feedback-in #8(w254) -> ()
                n134 = feedback #9(fxp<+/-,16,1> 0.0 ("Trap Pos FB Int-Norm Signal")) -> (w237:fxp<+/-,16,1>)
                n135 = Select(t=w235, s=w234, f=w237) -> (s? t:f=w236:fxp<+/-,16,1>)
                "Trap Pos FB Int-Norm Signal" <- w236
                n136 = feedback-in #9(w236) -> ()
                n137 = case "For position feedback" shown="True" "Force feedback" {
                  tunnel: [i64 0 w295] -> w255
                  tunnel: w235 -> [_ w292]
                  tunnel: w234 -> [_ w291]
                  frame False {
                  }
                  frame True {
                    n138 = feedback #10(i64 0) -> (w294:i64)
                    n139 = case shown="True" w291 {
                      tunnel: [w296 w310] -> w295
                      tunnel: w294 -> [w296 _]
                      tunnel: w292 -> [_ w304]
                      frame False {
                      }
                      frame True {
                        w314 = u32 0
                        n140 = Bundle("P2"="P2", "I2"="I2", "D2"="D2") -> (w300:T8)  [unwired: 1 in]
                        n141 = Bundle("FB2 output high"="FB2 output high", "FB2 output low"="FB2 output low") -> (w297:T9)  [unwired: 1 in]
                        n142 = xnode ("PID")("process variable"=w304, "reset?"="Trap Pos. FB Reset", "setpoint"="Trap Pos. FB SP", "PID gains"=w300, "output range"=w297) -> ("output"=w326:fxp<+/-,16,1>)
                        n143 = Negate(x=w326) -> (-x=w325:fxp<+/-,17,2>)
                        n144 = Select(t=w325, s="Trap Pos FB Negate Action", f=w326) -> (s? t:f=w322:fxp<+/-,17,2>)
                        n145 = Scale By Power Of 2(n=u32 15, x=u32 1) -> (x*2^n=w319:u32)
                        n146 = Multiply(x=w322, y=w319) -> (x*y=w318:fxp<+/-,17,17>)
                        n147 = To Quad Integer(1:w318) -> (0:w330:i64)
                        "Trap Pos FB Action" <- w330
                        n148 = Multiply(x=w330, y="Trap Pos. FB Mult Factor") -> (x*y=w328:i64)
                        n149 = Add(x=w328, y="Trap Pos. FB Offset Factor") -> (x+y=w310:i64)
                        n150 = feedback #11() -> (w311:i64)  [unwired: 1 in]
                        n151 = Add(x=w310, y=w311) -> (x+y=w308:i64)
                        n152 = feedback #12(w314) -> (w316:u32)
                        n153 = Increment(x=w316) -> (x+1=w305:u32)
                        n154 = Greater Or Equal?(x=w305, y="FB Trig Integrate") -> (x >= y?=w306:bool)
                        n155 = Select(t=i64 0, s=w306, f=w308) -> (s? t:f=w312:i64)
                        n156 = feedback-in #11(w312) -> ()
                        n157 = Select(t=w314, s=w306, f=w305) -> (s? t:f=w315:u32)
                        n158 = feedback-in #12(w315) -> ()
                        n159 = And(x=w306, y="FPGA Trap Trig") -> (x .and. y?=w313:bool)
                        n160 = case "Trap FB trigger excitation laser ON" shown="True" w313 {
                          tunnel: w308 -> [_ w334]
                          tunnel: w305 -> [_ w332]
                          frame False {
                          }
                          frame True {
                            n161 = Not(x="TTrig Negate Pos") -> (.not. x?=w341:bool)
                            n162 = Boolean To (0,1)(Boolean="TTrig Negate Pos") -> (0, 1=w339:i16)
                            n163 = Boolean To (0,1)(Boolean=w341) -> (0, 1=w340:i16)
                            n164 = Negate(x=w339) -> (-x=w338:i16)
                            n165 = Add(x=w338, y=w340) -> (x+y=w337:i16)
                            n166 = Multiply(x=w337, y=w334) -> (x*y=w336:i64)
                            "TTrig Sig" <- w336
                            n167 = Multiply(x="FPGA TTrig Thresh", y=w332) -> (x*y=w333:i64)
                            "TTrig Fin Thresh" <- w333
                            n168 = Greater Or Equal?(x=w336, y=w333) -> (x >= y?=w335:bool)
                            n169 = case shown="True" w335 {
                              frame False {
                              }
                              frame True {
                                w344 = TRUE ("Green FB On/Off")
                                w346 = u8 2 ("Operating Mode")
                                n170 = local write "Operating Mode 2"(w346) -> ()
                                n171 = local write "Operating Mode"(w346) -> ()
                                n172 = local write "Green FB On/Off"(w344) -> ()
                                n173 = local write "FPGA Trap Trig"(FALSE ("FPGA Trap Trig")) -> ()
                                "TTrig?" <- w344
                              }
                            }
                          }
                        }
                      }
                    }
                    n174 = feedback-in #10(w295) -> ()
                  }
                }
                n175 = Select(t=w265, s="Scan BD", f=w266) -> (s? t:f=w264:u64)
                n176 = Select(t=w266, s="Scan BD", f=w265) -> (s? t:f=w267:u64)
                n177 = Add(x=w264, y="BD 2 Frequency 1") -> (x+y=w269:u64)
                n178 = Compound Arithmetic op=ADD("BD 1 Frequency 1", w255, w267) -> (w270:u64)
                "BD1 Frequency Out 1" <- w270
              }
              frame 2 {
                # "Trap 2"
                n179 = case shown="True" "FB On/Off Set 2" {
                  tunnel: [w433 w436] -> w429
                  tunnel: "BD 1 Amplitude 2" -> [w433 _]
                  tunnel: w426 -> [_ w435]
                  tunnel: w425 -> [_ w434]
                  frame False {
                  }
                  frame True {
                    n180 = local read "AI2 Y Sum Set 2"() -> (w439:i16)
                    n181 = call "Slower PID.vi"("process variable"=w439, "reset?"="FB Reset Set 2", "setpoint"="FB Setpoint Set 2", "PID gains (x 2^8)"=w435, "output range"=w434) -> ("output"=w437:i16)  [unwired: 10 out]
                    n182 = To Unsigned Word Integer(number=w437) -> (unsigned 16bit integer=w436:u16)
                  }
                }
                "BD1 Frequency Out 2" <- "BD 1 Frequency 2"
              }
              frame 3 {
                # "Fluorescence period"
              }
            }
            n183 = feedback-in #13(w144) -> ()
            n184 = feedback #13(w144) -> (w143:u16)
            n185 = Select(t=w146, s="Interlace ON/OFF", f="Interlace Off Parameters") -> (s? t:f=w184:u8)
            n186 = Subtract(x=w144, y=w143) -> (x-y=w142:u16)
            n187 = Subtract "The error"(x=w142, y=w141) -> (x-y=w119:u16)
            n188 = case shown="1, Default" w184 {
              tunnel: ["DIO count 1 (ticks)" "DIO count 2 (ticks)" "DIO count 3 (ticks)"] -> w140
              frame 1, Default {
              }
              frame 2 {
              }
              frame 3 {
              }
            }
            n189 = Number To Boolean Array(number=w119) -> (Boolean array=w120:bool[])
            n190 = Or Array Elements(Boolean array=w120) -> (logical OR=w118:bool)
            n191 = Boolean To (0,1)(Boolean=w118) -> (0, 1=w125:i16)
            n192 = To Unsigned Byte Integer(number=w125) -> (unsigned 8bit integer=w122:u8)
            n193 = feedback #14(u8 0) -> (w123:u8)
            n194 = Add(x=w122, y=w123) -> (x+y=w121:u8)
            "DIO Late Counter" <- w121
            n195 = feedback-in #14(w121) -> ()
            n196 = Subtract(x=w140, y=w119) -> (x-y=w139:u16)
            n197 = Split Number(x=w181) -> (hi(x)=w180:u32, lo(x)=w179:u32)
            n198 = Split Number(x=w170) -> (hi(x)=w175:u32, lo(x)=w174:u32)
            n199 = Boolean To (0,1)(Boolean="+ phase (DIO)") -> (0, 1=w136:i16)
            n200 = Split Number(x=w180) -> (lo(x)=w178:u16)  [unwired: 1 out]
            n201 = Split Number(x=w179) -> (hi(x)=w177:u16, lo(x)=w176:u16)
            n202 = Split Number(x=w175) -> (lo(x)=w173:u16)  [unwired: 1 out]
            n203 = Split Number(x=w174) -> (hi(x)=w172:u16, lo(x)=w171:u16)
            n204 = Split Number(x=w129) -> (hi(x)=w131:u8, lo(x)=w130:u8)
            n205 = Split Number(x=w126) -> (hi(x)=w128:u8, lo(x)=w127:u8)
            n206 = Split Number(x=w178) -> (hi(x)=w168:u8, lo(x)=w167:u8)
            n207 = Split Number(x=w177) -> (hi(x)=w166:u8, lo(x)=w165:u8)
            n208 = Split Number(x=w173) -> (hi(x)=w161:u8, lo(x)=w160:u8)
            n209 = Split Number(x=w176) -> (hi(x)=w164:u8, lo(x)=w163:u8)
            n210 = Split Number(x=w172) -> (hi(x)=w159:u8, lo(x)=w158:u8)
            n211 = Split Number(x=w171) -> (hi(x)=w157:u8, lo(x)=w156:u8)
            n212 = Multiply(x=w136, y="Phase count adjustment (DIO)") -> (x*y=w132:i16)
            n213 = feedback #15(i16 0) -> (w134:i16)
            n214 = Subtract(x=w134, y=w132) -> (x-y=w133:i16)
            "DIO Relative phase" <- w133
            n215 = feedback-in #15(w133) -> ()
            n216 = Add(x=w139, y=w132) -> (x+y=w138:u16)
            n217 = Build Array "BD 1 A Stack"(w131, w130) -> (w153:u8[])
            n218 = Build Array "BD 2 A Stack"(w128, w127) -> (w152:u8[])
            n219 = Build Array "BD 1 nu Stack"(w168, w167, w166, w165, w164, w163) -> (w162:u8[])
            n220 = Build Array "BD 2 nu Stack"(w161, w160, w159, w158, w157, w156) -> (w155:u8[])
            n221 = case shown="2" w169 {
              tunnel: [w224 w227] -> w151
              tunnel: [u8 10 u8 4] -> w154
              tunnel: "Swap F1 and F2" -> [w225 w227]
              frame 2 {
                # "F2"
                n222 = Not(x=w225) -> (.not. x?=w224:bool)
              }
              frame 1, Default {
                # "low chooses F1"
                # "F1"
              }
            }
            n223 = case "If FPGA is controlling (toggling) RF synth" shown="True" w150 {
              tunnel: w162 -> [_ w200]
              tunnel: w155 -> [_ w199]
              tunnel: w154 -> [_ w198]
              tunnel: w153 -> [_ w197]
              tunnel: w152 -> [_ w196]
              frame False {
              }
              frame True {
                # "Write next amp.\n(wait until beginning of next loop iteration to update)"
                n224 = flat-sequence "Update the next F1 and F2 frequency value (the actual frequency won't change until FSK is switched).\nThen load the next amplitude value into buffer, but don't update it until the next cycle." {
                  tunnel: w199 -> [w202]
                  tunnel: w200 -> [w203]
                  tunnel: [w203] -> w195
                  tunnel: [w202] -> w194
                  tunnel: w198 -> [w204]
                  tunnel: w195 -> [w206]
                  tunnel: w194 -> [w205]
                  tunnel: w197 -> [w217]
                  tunnel: w196 -> [w216]
                  frame #0 {
                    # "To possibly send\nthese writes to very\nend of loop (for x and\ny phase adjust)"
                    n225 = call "Wait8"("Count(Ticks)"="Next trap write delay (ticks)") -> ()  [unwired: 1 out]
                  }
                  frame #1 {
                    n226 = for {
                      tunnel: w206 -> [w212] mode=indexing
                      tunnel: w205 -> [w211] mode=indexing
                      tunnel: w204 -> [w209]
                      i -> [w210]
                      # "Write next freq."
                      n227 = To Unsigned Byte Integer(number=w210) -> (unsigned 8bit integer=w207:u8)
                      n228 = Add(x=w209, y=w207) -> (x+y=w208:u8)
                      n229 = call "write to RF synth bd.vi"("Address Byte"=w208, "BD 2 Byte"=w211, "BD 1 Byte"=w212) -> ()
                    }
                  }
                  frame #2 {
                    w213 = TRUE ("Connector1/DIO15")
                    # "send udclk high\n(BD 1 and 2)"
                    n230 = xnode "FPGA I/O Node"("Connector1/DIO30"=w213, "Connector1/DIO29"=w213) -> ()  [unwired: 2 in, 2 out]
                  }
                  frame #3 {
                    w214 = FALSE ("Connector1/DIO15")
                    n231 = xnode "FPGA I/O Node"("Connector1/DIO30"=w214, "Connector1/DIO29"=w214) -> ()  [unwired: 2 in, 2 out]
                  }
                  frame #4 {
                    n232 = for {
                      tunnel: w217 -> [w223] mode=indexing
                      tunnel: w216 -> [w222] mode=indexing
                      tunnel: u8 33 -> [w220]
                      i -> [w221]
                      n233 = To Unsigned Byte Integer(number=w221) -> (unsigned 8bit integer=w218:u8)
                      n234 = Add(x=w220, y=w218) -> (x+y=w219:u8)
                      n235 = call "write to RF synth bd.vi"("Address Byte"=w219, "BD 2 Byte"=w222, "BD 1 Byte"=w223) -> ()
                    }
                  }
                }
              }
            }
          }
        }
      }
    }
  }
  n236 = while "RF box board direct communication loop" {
    tunnel: w1 -> [_]
    stop <- FALSE stop-if-true
    n237 = case "Whether to use direct communication method (only use one method at a time)" shown="True" "Direct RF Box \nCommunication" {
      frame False {
      }
      frame True {
        n238 = case shown="True" "Update Data" {
          frame False {
          }
          frame True {
            n239 = flat-sequence {
              frame #0 {
                n240 = First Call?() -> (First Call?: T/F=w448:bool)
                n241 = case shown="True" w448 {
                  frame False {
                  }
                  frame True {
                    # "If first time data updated, be sure to set WR high\nbefore setting data and address bits."
                    n242 = flat-sequence {
                      frame #0 {
                        n243 = xnode "FPGA I/O Node"("Connector1/DIO15"=TRUE) -> ()  [unwired: 1 in, 1 out]
                      }
                      frame #1 {
                        n244 = call "Wait"("Count(Ticks)"=u8 40 ("DO Delay 3 (Ticks)")) -> ()  [unwired: 1 out]
                      }
                    }
                  }
                }
              }
              frame #1 {
                n245 = Number To Boolean Array(number="Address") -> (Boolean array=w497:bool[])
                n246 = Number To Boolean Array(number="Data BD 1") -> (Boolean array=w498:bool[])
                n247 = Number To Boolean Array(number="Data BD 2") -> (Boolean array=w467:bool[])
                n248 = Index Array(array=w498, index=7) -> (element=w482:bool)
                n249 = Index Array(array=w498, index=6) -> (element=w481:bool)
                n250 = Index Array(array=w498, index=5) -> (element=w480:bool)
                n251 = Index Array(array=w498, index=4) -> (element=w479:bool)
                n252 = Index Array(array=w498, index=3) -> (element=w478:bool)
                n253 = Index Array(array=w498, index=2) -> (element=w477:bool)
                n254 = Index Array(array=w498, index=1) -> (element=w476:bool)
                n255 = Index Array(array=w498, index=0) -> (element=w475:bool)
                n256 = Index Array(array=w497, index=5) -> (element=w474:bool)
                n257 = Index Array(array=w497, index=4) -> (element=w473:bool)
                n258 = Index Array(array=w497, index=3) -> (element=w472:bool)
                n259 = Index Array(array=w497, index=2) -> (element=w471:bool)
                n260 = Index Array(array=w497, index=1) -> (element=w470:bool)
                n261 = Index Array(array=w497, index=0) -> (element=w469:bool)
                n262 = Index Array(array=w467, index=7) -> (element=w458:bool)
                n263 = Index Array(array=w467, index=6) -> (element=w457:bool)
                n264 = Index Array(array=w467, index=5) -> (element=w456:bool)
                n265 = Index Array(array=w467, index=4) -> (element=w455:bool)
                n266 = Index Array(array=w467, index=3) -> (element=w454:bool)
                n267 = Index Array(array=w467, index=2) -> (element=w453:bool)
                n268 = Index Array(array=w467, index=1) -> (element=w452:bool)
                n269 = Index Array(array=w467, index=0) -> (element=w451:bool)
                n270 = xnode "FPGA I/O Node"("Connector1/DIO0"=w482, "Connector1/DIO1"=w481, "Connector1/DIO2"=w480, "Connector1/DIO3"=w479, "Connector1/DIO4"=w478, "Connector1/DIO5"=w477, "Connector1/DIO6"=w476, "Connector1/DIO7"=w475, "Connector1/DIO8"=w474, "Connector1/DIO9"=w473, "Connector1/DIO10"=w472, "Connector1/DIO11"=w471, "Connector1/DIO12"=w470, "Connector1/DIO13"=w469, "Connector1/DIO20"=w458, "Connector1/DIO21"=w457, "Connector1/DIO22"=w456, "Connector1/DIO23"=w455, "Connector1/DIO24"=w454, "Connector1/DIO25"=w453, "Connector1/DIO26"=w452, "Connector1/DIO27"=w451) -> ()  [unwired: 22 in, 22 out]
              }
              frame #2 {
                # "wait and then apply write signal"
                n271 = call "Wait2"("Count(Ticks)"=u8 40 ("DO Delay 1 (Ticks)")) -> ()  [unwired: 1 out]
              }
              frame #3 {
                # "sending bit low writes data to board buffer"
                n272 = xnode "FPGA I/O Node"("Connector1/DIO15"=FALSE) -> ()  [unwired: 1 in, 1 out]
              }
              frame #4 {
                # "wait then return write signal"
                n273 = call "Wait3"("Count(Ticks)"=u8 40 ("DO Delay 2 (Ticks)")) -> ()  [unwired: 1 out]
              }
              frame #5 {
                # "sending bit high makes ready to\nwrite more data"
                n274 = xnode "FPGA I/O Node"("Connector1/DIO15"=TRUE) -> ()  [unwired: 1 in, 1 out]
              }
            }
          }
        }
      }
    }
  }
  n275 = To Unsigned Long Integer(number=w1) -> (unsigned 32bit integer=w6:u32)
  n276 = while "APD 1 Counter" {
    tunnel: w1 -> [_]
    stop <- FALSE stop-if-true
    n277 = flat-sequence {
      frame #0 {
        n278 = xnode "FPGA I/O Method Node"("FPGA I/O In"=refnum<k21> "Connector0/DIO0" ("APD 1 DO"), "Timeout"=-1) -> ()  [unwired: 2 out]
      }
      frame #1 {
        n279 = local read "APD1 out state"() -> (w508:bool)
        n280 = case shown="False" w508 {
          frame False {
            n281 = local read "APD 1 Counts 0"() -> (w510:u32)
            n282 = Increment(x=w510) -> (x+1=→"APD 1 Counts 0":u32)
          }
          frame True {
            n283 = local read "APD 1 Counts 1"() -> (w512:u32)
            n284 = Increment(x=w512) -> (x+1=→"APD 1 Counts 1":u32)
          }
        }
      }
    }
  }
  n285 = while "APD 2 Counter" {
    tunnel: w1 -> [_]
    stop <- FALSE stop-if-true
    n286 = flat-sequence {
      frame #0 {
        n287 = xnode "FPGA I/O Method Node"("FPGA I/O In"=refnum<k21> "Connector0/DIO1" ("APD 2 DO"), "Timeout"=-1) -> ()  [unwired: 2 out]
      }
      frame #1 {
        n288 = local read "APD2 out state"() -> (w516:bool)
        n289 = case shown="False" w516 {
          frame False {
            n290 = local read "APD 2 Counts 0"() -> (w518:u32)
            n291 = Increment(x=w518) -> (x+1=→"APD 2 Counts 0":u32)
          }
          frame True {
            n292 = local read "APD 2 Counts 1"() -> (w520:u32)
            n293 = Increment(x=w520) -> (x+1=→"APD 2 Counts 1":u32)
          }
        }
      }
    }
  }
  n294 = while "APD 2 Gating" {
    shift-right: [w524] -> _
    shift-left: w1 -> [w529]
    shift-right: [w523] -> _
    shift-left: w5 -> [w521]
    stop <- FALSE stop-if-true
    n295 = flat-sequence {
      tunnel: w529 -> [w532]
      tunnel: [w533] -> w527
      tunnel: [w532] -> w525
      tunnel: [w531] -> w522
      tunnel: w521 -> [w531]
      tunnel: [w536] -> w528
      tunnel: w527 -> [w536]
      tunnel: [w535] -> w526
      tunnel: w525 -> [w535]
      tunnel: w522 -> [w534]
      tunnel: [w554] -> w524
      tunnel: w528 -> [w565]
      tunnel: w526 -> [w563]
      tunnel: [w558] -> w523
      frame #0 {
        n296 = call "Loop Timer8"("Count(Ticks)"=w532) -> ("Tick Count(Ticks)"=w533:u16)
      }
      frame #1 {
        # "Signal is then sent through \na transistor before APD"
        n297 = xnode "FPGA I/O Node"("Connector0/DIO8"=w534) -> ()  [unwired: 1 in, 1 out]
      }
      frame #2 {
        n298 = local read "APD Gate ON Count"() -> (w547:u16)
        n299 = local read "APD Gate OFF Count"() -> (w546:u16)
        n300 = feedback #16(TRUE) -> (w560:bool)
        n301 = feedback-in #17(w565) -> ()
        n302 = feedback #17(w565) -> (w548:u16)
        n303 = Not(x=w560) -> (.not. x?=w557:bool)
        n304 = feedback-in #16(w557) -> ()
        n305 = Subtract(x=w565, y=w548) -> (x-y=w564:u16)
        n306 = Select(t=w547, s=w557, f=w546) -> (s? t:f=w562:u16)
        n307 = Subtract(x=w564, y=w563) -> (x-y=w539:u16)
        n308 = Subtract(x=w562, y=w539) -> (x-y=w553:u16)
        n309 = Number To Boolean Array(number=w539) -> (Boolean array=w538:bool[])
        n310 = Or Array Elements(Boolean array=w538) -> (logical OR=w537:bool)
        n311 = Boolean To (0,1)(Boolean="+ phase (APD 2 Gate)") -> (0, 1=w551:i16)
        n312 = Multiply(x=w551, y="Phase count adjustment (APD 2 Gate)") -> (x*y=w549:i16)
        n313 = Boolean To (0,1)(Boolean=w537) -> (0, 1=w544:i16)
        n314 = Add(x=w553, y=w549) -> (x+y=w554:u16)
        n315 = To Unsigned Byte Integer(number=w544) -> (unsigned 8bit integer=w541:u8)
        n316 = feedback #18(i16 0) -> (w556:i16)
        n317 = Subtract(x=w556, y=w549) -> (x-y=w555:i16)
        "APD 2 Gate Relative Phase" <- w555
        n318 = feedback-in #18(w555) -> ()
        n319 = feedback #19(u8 0) -> (w542:u8)
        n320 = Add(x=w541, y=w542) -> (x+y=w540:u8)
        "APD 2 Gate Late Counter" <- w540
        n321 = feedback-in #19(w540) -> ()
        n322 = local read "APD Gate Operating Mode"() -> (w545:u8)
        n323 = case shown="2" w545 {
          tunnel: [TRUE FALSE w571] -> w558
          tunnel: w560 -> [_ _ w569]
          frame 0, Default {
          }
          frame 1 {
          }
          frame 2 {
            n324 = local read "Invert APD Gate"() -> (w568:bool)
            n325 = Not(x=w569) -> (.not. x?=w570:bool)
            n326 = Select(t=w570, s=w568, f=w569) -> (s? t:f=w571:bool)
          }
        }
      }
    }
  }
  n327 = while "532 nm green fluorescent laser interlacing (DO to IA 532 nm AOM ME amp)." {
    shift-right: [w575] -> _
    shift-left: w1 -> [w580]
    shift-right: [w574] -> _
    shift-left: w2 -> [w572]
    stop <- FALSE stop-if-true
    n328 = flat-sequence {
      tunnel: w580 -> [w583]
      tunnel: [w584] -> w578
      tunnel: [w583] -> w576
      tunnel: [w582] -> w573
      tunnel: w572 -> [w582]
      tunnel: [w587] -> w579
      tunnel: w578 -> [w587]
      tunnel: [w586] -> w577
      tunnel: w576 -> [w586]
      tunnel: w573 -> [w585]
      tunnel: [w596] -> w575
      tunnel: w579 -> [w616]
      tunnel: w577 -> [w613]
      tunnel: [w605] -> w574
      frame #0 {
        n329 = call "Loop Timer4"("Count(Ticks)"=w583) -> ("Tick Count(Ticks)"=w584:u16)
      }
      frame #1 {
        # "Then to PRL 440 amp"
        n330 = xnode "FPGA I/O Node"("Connector1/DIO39"=w585) -> ()  [unwired: 1 in, 1 out]
      }
      frame #2 {
        n331 = feedback-in #20(w616) -> ()
        n332 = feedback #20(w616) -> (w615:u16)
        n333 = Subtract(x=w616, y=w615) -> (x-y=w614:u16)
        n334 = Subtract(x=w614, y=w613) -> (x-y=w589:u16)
        n335 = Number To Boolean Array(number=w589) -> (Boolean array=w590:bool[])
        n336 = Or Array Elements(Boolean array=w590) -> (logical OR=w588:bool)
        n337 = Boolean To (0,1)(Boolean="+ phase (GI)") -> (0, 1=w601:i16)
        n338 = Multiply(x=w601, y="Phase count adjustment (GI)") -> (x*y=w598:i16)
        n339 = Boolean To (0,1)(Boolean=w588) -> (0, 1=w595:i16)
        n340 = To Unsigned Byte Integer(number=w595) -> (unsigned 8bit integer=w592:u8)
        n341 = feedback #21(i16 0) -> (w599:i16)
        n342 = feedback #22(u8 0) -> (w593:u8)
        n343 = Add(x=w592, y=w593) -> (x+y=w591:u8)
        "GI Late Counter" <- w591
        n344 = feedback-in #22(w591) -> ()
        n345 = Subtract(x=w599, y=w598) -> (x-y=w597:i16)
        "GI Relative phase" <- w597
        n346 = feedback-in #21(w597) -> ()
        n347 = feedback #23(TRUE) -> (w608:bool)
        n348 = case shown="2" "Operating Mode" {
          tunnel: [TRUE FALSE w622] -> w605
          tunnel: w608 -> [_ _ w619]
          frame 0, Default {
          }
          frame 1 {
          }
          frame 2 {
            n349 = Not(x=w619) -> (.not. x?=w621:bool)
            n350 = Select(t=w621, s="Invert GI", f=w619) -> (s? t:f=w622:bool)
          }
        }
        n351 = Not(x=w608) -> (.not. x?=w604:bool)
        n352 = Select(t="Green interlace ON count", s=w604, f="Green interlace OFF count") -> (s? t:f=w610:u16)
        n353 = Subtract(x=w610, y=w589) -> (x-y=w602:u16)
        n354 = Add(x=w602, y=w598) -> (x+y=w596:u16)
        n355 = feedback-in #23(w604) -> ()
      }
    }
  }
  n356 = while "Green and red fluorescent laser interlacing (Current AO to IA 532 nm AOM ME amp)." {
    shift-right: [w631] -> _
    shift-left: w1 -> [w634]
    shift-right: [w628] -> _
    shift-left: w3 -> [w626]
    shift-right: [w625] -> _
    shift-left: w3 -> [w624]
    stop <- FALSE stop-if-true
    n357 = flat-sequence {
      tunnel: w634 -> [w638]
      tunnel: [w639] -> w633
      tunnel: [w638] -> w632
      tunnel: [w637] -> w627
      tunnel: w626 -> [w637]
      tunnel: w624 -> [w636]
      tunnel: [w636] -> w623
      tunnel: [w643] -> w630
      tunnel: w633 -> [w643]
      tunnel: [w642] -> w629
      tunnel: w632 -> [w642]
      tunnel: w627 -> [w641]
      tunnel: w623 -> [w640]
      tunnel: [w664] -> w631
      tunnel: [w680] -> w628
      tunnel: w630 -> [w691]
      tunnel: w629 -> [w688]
      tunnel: [w648] -> w625
      frame #0 {
        n358 = call "Loop Timer10"("Count(Ticks)"=w638) -> ("Tick Count(Ticks)"=w639:u16)
      }
      frame #1 {
        n359 = xnode "FPGA I/O Node"("Chassis2/Mod4/AO0"=w641, "Chassis2/Mod4/AO1"=w640) -> ()  [unwired: 2 in, 2 out]
      }
      frame #2 {
        # "Design note:\n\nThese two laser controls are in the same loop\nbecause the expansion current AI cannot separately\ntime the outputs fast enough for us.  Apparently\nit is because of communication time between the\nexpansion card and the fpga.\n\nSo the two analog control signals have the same timing\nand profile, but independent amplitudes to independently\ncontrol the intensity and feedback for each laser."
        n360 = feedback #24(TRUE) -> (w644:bool)
        n361 = Not(x=w644) -> (.not. x?=w645:bool)
        n362 = feedback-in #24(w645) -> ()
        n363 = Subtract(x="Green interlace OFF count 2", y="Green int current ON count adj") -> (x-y=w673:u16)
        n364 = feedback-in #25(w691) -> ()
        n365 = feedback #25(w691) -> (w690:u16)
        n366 = Add(x="Green int current ON count adj", y="Green interlace ON count 2") -> (x+y=w674:u16)
        n367 = Subtract(x=w691, y=w690) -> (x-y=w689:u16)
        n368 = Select(t=w674, s=w645, f=w673) -> (s? t:f=w685:u16)
        n369 = Subtract(x=w689, y=w688) -> (x-y=w657:u16)
        n370 = case shown="2" "RI Operating Mode 2" {
          tunnel: [TRUE FALSE w697] -> w646
          tunnel: w644 -> [_ _ w694]
          frame 0, Default {
          }
          frame 1 {
          }
          frame 2 {
            n371 = Not(x=w694) -> (.not. x?=w696:bool)
            n372 = Select(t=w696, s="Invert RI 2", f=w694) -> (s? t:f=w697:bool)
          }
        }
        n373 = Subtract(x=w685, y=w657) -> (x-y=w668:u16)
        n374 = case shown="0, Default" "Operating Mode 2" {
          tunnel: [TRUE FALSE w731] -> w649
          tunnel: w644 -> [_ _ w728]
          frame 0, Default {
          }
          frame 1 {
          }
          frame 2 {
            n375 = Not(x=w728) -> (.not. x?=w730:bool)
            n376 = Select(t=w730, s="Invert GI 2", f=w728) -> (s? t:f=w731:bool)
          }
        }
        n377 = Number To Boolean Array(number=w657) -> (Boolean array=w658:bool[])
        n378 = Boolean To (0,1)(Boolean="+ phase (GI) 2") -> (0, 1=w670:i16)
        n379 = Or Array Elements(Boolean array=w658) -> (logical OR=w656:bool)
        n380 = Boolean To (0,1)(Boolean=w656) -> (0, 1=w663:i16)
        n381 = Multiply(x=w670, y="Phase count adjustment (GI) 2") -> (x*y=w666:i16)
        n382 = To Unsigned Byte Integer(number=w663) -> (unsigned 8bit integer=w659:u8)
        n383 = Add(x=w668, y=w666) -> (x+y=w664:u16)
        n384 = feedback #26(u8 0) -> (w661:u8)
        n385 = Add(x=w659, y=w661) -> (x+y=w660:u8)
        "GI Late Counter 2" <- w660
        n386 = feedback-in #26(w660) -> ()
        n387 = feedback #27(i16 0) -> (w667:i16)
        n388 = Subtract(x=w667, y=w666) -> (x-y=w665:i16)
        "GI Relative phase 2" <- w665
        n389 = feedback-in #27(w665) -> ()
        n390 = And(x=w649, y="Green FB On/Off") -> (x .and. y?=w675:bool)
        n391 = And(x=w646, y="Red FB On/Off") -> (x .and. y?=w655:bool)
        n392 = case shown="True" w675 {
          tunnel: "Current Out" -> [w712 _]
          tunnel: [w712 w721] -> w679
          frame False {
          }
          frame True {
            n393 = local read "Green FB Sum"() -> (w717:i16)
            n394 = Bundle("P3"="P3", "I3"="I3", "D3"="D3") -> (w713:cluster{"P3":i16, "I3":i16, "D3":i16})  [unwired: 1 in]
            n395 = call "Slower PID.vi"("process variable"=w717, "reset?"="Green FB Reset", "setpoint"="Green FB Setpoint", "PID gains (x 2^8)"=w713, "output range"=cluster{"output high":i16, "output low":i16} {"output high"=32767, "output low"=-32768} ("Green FB output range")) -> ("output"=w724:i16)  [unwired: 10 out]
            n396 = To Long Integer(number=w724) -> (32bit integer=w718:i32)
            n397 = Add(x=w718, y=32768) -> (x+y=w720:i32)
            n398 = To Unsigned Word Integer(number=w720) -> (unsigned 16bit integer=w721:u16)
          }
        }
        n399 = case shown="True" w655 {
          tunnel: "RI Current Out" -> [w698 _]
          tunnel: [w698 w707] -> w651
          frame False {
          }
          frame True {
            n400 = local read "Red FB Intensity"() -> (w703:i16)
            n401 = Bundle("P4"="P4", "I4"="I4", "D4"="D4") -> (w699:cluster{"P4":i16, "I4":i16, "D4":i16})  [unwired: 1 in]
            n402 = call "Slower PID.vi"("process variable"=w703, "reset?"="Red FB Reset", "setpoint"="Red FB Setpoint", "PID gains (x 2^8)"=w699, "output range"=cluster{"output high":i16, "output low":i16} {"output high"=32767, "output low"=-32768} ("Green FB output range")) -> ("output"=w710:i16)  [unwired: 10 out]
            n403 = To Long Integer(number=w710) -> (32bit integer=w704:i32)
            n404 = Add(x=w704, y=32768) -> (x+y=w706:i32)
            n405 = To Unsigned Word Integer(number=w706) -> (unsigned 16bit integer=w707:u16)
          }
        }
        n406 = Boolean To (0,1)(Boolean=w649) -> (0, 1=w681:i16)
        n407 = Boolean To (0,1)(Boolean=w646) -> (0, 1=w650:i16)
        n408 = To Unsigned Word Integer(number=w681) -> (unsigned 16bit integer=w678:u16)
        n409 = To Unsigned Word Integer(number=w650) -> (unsigned 16bit integer=w652:u16)
        n410 = Multiply(x=w678, y=w679) -> (x*y=w680:u16)
        n411 = Multiply(x=w652, y=w651) -> (x*y=w648:u16)
      }
    }
  }
  n412 = while "MCL stage control" {
    shift-right: [w744] -> _
    shift-left: w1 -> [w747]
    shift-right: [w737] -> _
    shift-left: w10 -> [w734]
    shift-right: [w736] -> _
    shift-left: w9 -> [w732]
    stop <- FALSE stop-if-true
    n413 = flat-sequence {
      tunnel: w747 -> [w751]
      tunnel: [w752] -> w743
      tunnel: [w751] -> w741
      tunnel: [w750] -> w735
      tunnel: w734 -> [w750]
      tunnel: [w749] -> w733
      tunnel: w732 -> [w749]
      tunnel: w743 -> [w756]
      tunnel: [w756] -> w742
      tunnel: w741 -> [w755]
      tunnel: [w755] -> w740
      tunnel: w735 -> [w754]
      tunnel: w733 -> [w753]
      tunnel: w742 -> [w764]
      tunnel: w740 -> [w763]
      tunnel: [w764] -> w746
      tunnel: [w763] -> w745
      tunnel: [w762] -> w739
      tunnel: [w761] -> w738
      tunnel: [w836] -> w744
      tunnel: w746 -> [w843]
      tunnel: w745 -> [w840]
      tunnel: w739 -> [w838]
      tunnel: w738 -> [w837]
      tunnel: [w838] -> w737
      tunnel: [w837] -> w736
      frame #0 {
        n414 = call "Loop Timer5"("Count(Ticks)"=w751) -> ("Tick Count(Ticks)"=w752:u32)
      }
      frame #1 {
        n415 = xnode "FPGA I/O Node"("Connector0/AO1"=w754, "Connector0/AO2"=w753) -> ()  [unwired: 2 in, 2 out]
      }
      frame #2 {
        n416 = local read "Scanning MCL"() -> (w776:bool)
        n417 = Or(x=w776, y="Start scan (MCL)") -> (x .or. y?=w771:bool)
        n418 = Not(x="Abort scan (MCL)") -> (.not. x?=w769:bool)
        n419 = And(x=w769, y=w771) -> (x .and. y?=w768:bool)
        n420 = case "Raster scan" shown="True" w768 {
          tunnel: [w777 w820] -> w773
          tunnel: "Start scan (MCL)" -> [_ w805]
          tunnel: [w777 w781] -> w757
          frame False {
            w777 = i16 0
            n421 = local write "Scanning MCL"(FALSE ("scanning")) -> ()
          }
          frame True {
            w791 = i16 0
            w790 = u64 0
            # "scan incr."
            # "freq. incr. mult."
            # "count steps"
            # "count number of cycles"
            n422 = feedback #28(w790) -> (w817:u64)
            n423 = Select(t=w790, s=w805, f=w817) -> (s? t:f=w819:u64)
            n424 = Increment(x=w819) -> (x+1=w816:u64)
            n425 = Greater?(x="Cycles per step (MCL)", y=w816) -> (0:w800:bool)
            n426 = Select(t=w816, s=w800, f=w790) -> (s? t:f=w815:u64)
            n427 = feedback-in #28(w815) -> ()
            n428 = feedback #29(w790) -> (w814:u64)
            n429 = Select(t=w790, s=w805, f=w814) -> (s? t:f=w809:u64)
            n430 = Increment(x=w809) -> (x+1=w813:u64)
            n431 = Add(x="Scan steps (MCL)", y="Scan steps (MCL)") -> (x+y=w812:u64)
            n432 = Select(t=w809, s=w800, f=w813) -> (s? t:f=w795:u64)
            n433 = Greater?(x=w812, y=w795) -> (0:w794:bool)
            n434 = Select(t=w795, s=w794, f=w790) -> (s? t:f=w810:u64)
            n435 = feedback-in #29(w810) -> ()
            n436 = Equal?(x="Scan steps (MCL)", y=w795) -> (x = y?=w799:bool)
            n437 = Greater?(x="Scan steps (MCL)", y=w809) -> (0:w808:bool)
            n438 = feedback #30(w791) -> (w811:i16)
            n439 = Select(t=w791, s=w805, f=w811) -> (s? t:f=w797:i16)
            n440 = Increment(x=w797) -> (x+1=w807:i16)
            n441 = Decrement(x=w797) -> (x-1=w806:i16)
            n442 = Select(t=w807, s=w808, f=w806) -> (s? t:f=w798:i16)
            n443 = Select(t=w797, s=w799, f=w798) -> (s? t:f=w796:i16)
            n444 = Select(t=w797, s=w800, f=w796) -> (s? t:f=w792:i16)
            n445 = Select(t=w792, s=w794, f=w791) -> (s? t:f=w793:i16)
            n446 = feedback-in #30(w793) -> ()
            n447 = feedback #31(w790) -> (w804:u64)
            n448 = Select(t=w790, s=w805, f=w804) -> (s? t:f=w779:u64)
            n449 = Increment(x=w779) -> (x+1=w801:u64)
            n450 = Select(t=w779, s=w794, f=w801) -> (s? t:f=w780:u64)
            n451 = Greater?(x="Number of scans (MCL)", y=w780) -> (0:w787:bool)
            n452 = Multiply(x="Scan freq.  increment (MCL)", y=w797) -> (x*y=w820:i16)
            n453 = Select(t=TRUE, s="Cont. Scan (MCL)", f=w787) -> (s? t:f=w786:bool)
            "Scanning MCL" <- w786
            n454 = Select(t=w780, s=w786, f=w790) -> (s? t:f=w802:u64)
            n455 = feedback-in #31(w802) -> ()
            n456 = Increment(x=w780) -> (x+1=→"Scan I (MCL)":u64)
            n457 = To Word Integer(number=w779) -> (16bit integer=w782:i16)
            n458 = Multiply(x=w782, y="Scan freq.  increment (MCL)") -> (x*y=w781:i16)
          }
        }
        n459 = Select(t=w757, s="1D or 2D Scan?", f=i16 0) -> (s? t:f=w758:i16)
        n460 = Select(t=w758, s="MCL Scan Axis", f=w773) -> (s? t:f=w772:i16)
        n461 = Select(t=w773, s="MCL Scan Axis", f=w758) -> (s? t:f=w774:i16)
        n462 = Add(x=w772, y="AO2") -> (x+y=w761:i16)
        n463 = Add(x="AO1", y=w774) -> (x+y=w762:i16)
      }
      frame #3 {
        n464 = feedback-in #32(w843) -> ()
        n465 = feedback #32(w843) -> (w842:u32)
        n466 = Boolean To (0,1)(Boolean="+ phase (MCL)") -> (0, 1=w834:i16)
        n467 = Subtract(x=w843, y=w842) -> (x-y=w841:u32)
        n468 = Multiply(x=w834, y="Phase count adjustment (MCL)") -> (x*y=w830:i16)
        n469 = Subtract(x=w841, y=w840) -> (x-y=w822:u32)
        n470 = Subtract(x="MCL count", y=w822) -> (x-y=w832:u32)
        n471 = feedback #33(i16 0) -> (w831:i16)
        n472 = Subtract(x=w831, y=w830) -> (x-y=w829:i16)
        "MCL Relative Phase" <- w829
        n473 = feedback-in #33(w829) -> ()
        n474 = Number To Boolean Array(number=w822) -> (Boolean array=w823:bool[])
        n475 = Or Array Elements(Boolean array=w823) -> (logical OR=w821:bool)
        n476 = Boolean To (0,1)(Boolean=w821) -> (0, 1=w828:i16)
        n477 = Add(x=w832, y=w830) -> (x+y=w836:u32)
        n478 = To Unsigned Byte Integer(number=w828) -> (unsigned 8bit integer=w825:u8)
        n479 = feedback #34(u8 0) -> (w826:u8)
        n480 = Add(x=w825, y=w826) -> (x+y=w824:u8)
        "MCL Late Counter" <- w824
        n481 = feedback-in #34(w824) -> ()
      }
    }
  }
  n482 = while "Excitation laser intensity feedback measurement (all lasers)" {
    shift-right: [w845] -> _
    shift-left: w1 -> [w850]
    stop <- FALSE stop-if-true
    n483 = flat-sequence {
      tunnel: w850 -> [w852]
      tunnel: [w853] -> w848
      tunnel: [w852] -> w846
      tunnel: [w859] -> w849
      tunnel: w848 -> [w859]
      tunnel: [w858] -> w847
      tunnel: w846 -> [w858]
      tunnel: [w871] -> w845
      tunnel: w849 -> [w882]
      tunnel: w847 -> [w879]
      frame #0 {
        n484 = call "Loop Timer9"("Count(Ticks)"=w852) -> ("Tick Count(Ticks)"=w853:u16)
      }
      frame #1 {
        # "Design note:\n\nAll lasers need to be measured at the same \ntime because the AI expansion module\ncannot independently time the measurements\nwithin our requirements: their is dead time.\n\nThis probably wouldn't be an issue with the built\nin AI on the fpga board itself."
        n485 = xnode "FPGA I/O Node"("Connector1/DIO35"=TRUE) -> ("Chassis2/Mod1/AI2"=→"Blue Intensity":i16, "Chassis2/Mod1/AI1"=→"Red FB Intensity":i16, "Chassis2/Mod1/AI0"=→"Green FB Sum":i16)  [unwired: 4 in, 4 out]
      }
      frame #2 {
        n486 = feedback-in #35(w882) -> ()
        n487 = feedback #35(w882) -> (w881:u16)
        n488 = Subtract(x=w882, y=w881) -> (x-y=w880:u16)
        n489 = xnode "FPGA I/O Node"("Connector1/DIO35"=FALSE) -> ()  [unwired: 1 in, 1 out]
        n490 = Subtract(x=w880, y=w879) -> (x-y=w861:u16)
        n491 = Subtract(x="Green FB Count", y=w861) -> (x-y=w875:u16)
        n492 = Number To Boolean Array(number=w861) -> (Boolean array=w862:bool[])
        n493 = Or Array Elements(Boolean array=w862) -> (logical OR=w860:bool)
        n494 = Boolean To (0,1)(Boolean="+ phase (Green FB)") -> (0, 1=w873:i16)
        n495 = Boolean To (0,1)(Boolean=w860) -> (0, 1=w867:i16)
        n496 = Multiply(x=w873, y="Phase count adjustment (Green FB)") -> (x*y=w868:i16)
        n497 = Add(x=w875, y=w868) -> (x+y=w871:u16)
        n498 = To Unsigned Byte Integer(number=w867) -> (unsigned 8bit integer=w864:u8)
        n499 = feedback #36(i16 0) -> (w870:i16)
        n500 = Subtract(x=w870, y=w868) -> (x-y=w869:i16)
        "Green FB Relative Phase" <- w869
        n501 = feedback-in #36(w869) -> ()
        n502 = feedback #37(u8 0) -> (w865:u8)
        n503 = Add(x=w864, y=w865) -> (x+y=w863:u8)
        "Green Late Counter" <- w863
        n504 = feedback-in #37(w863) -> ()
      }
    }
  }
  n505 = while "APD 1 Gating" {
    shift-right: [w886] -> _
    shift-left: w1 -> [w891]
    shift-right: [w885] -> _
    shift-left: w5 -> [w883]
    stop <- FALSE stop-if-true
    n506 = flat-sequence {
      tunnel: w891 -> [w894]
      tunnel: [w895] -> w889
      tunnel: [w894] -> w887
      tunnel: [w893] -> w884
      tunnel: w883 -> [w893]
      tunnel: [w898] -> w890
      tunnel: w889 -> [w898]
      tunnel: [w897] -> w888
      tunnel: w887 -> [w897]
      tunnel: w884 -> [w896]
      tunnel: [w912] -> w886
      tunnel: w890 -> [w927]
      tunnel: w888 -> [w924]
      tunnel: [w916] -> w885
      frame #0 {
        n507 = call "Loop Timer7"("Count(Ticks)"=w894) -> ("Tick Count(Ticks)"=w895:u16)
      }
      frame #1 {
        # "Signal is then sent through \na transistor before APD"
        n508 = xnode "FPGA I/O Node"("Connector0/DIO4"=w896) -> ()  [unwired: 1 in, 1 out]
      }
      frame #2 {
        n509 = feedback #38(TRUE) -> (w919:bool)
        n510 = feedback-in #39(w927) -> ()
        n511 = feedback #39(w927) -> (w926:u16)
        n512 = Not(x=w919) -> (.not. x?=w915:bool)
        n513 = feedback-in #38(w915) -> ()
        n514 = Subtract(x=w927, y=w926) -> (x-y=w925:u16)
        n515 = Select(t="APD Gate ON Count", s=w915, f="APD Gate OFF Count") -> (s? t:f=w921:u16)
        n516 = Subtract(x=w925, y=w924) -> (x-y=w900:u16)
        n517 = Subtract(x=w921, y=w900) -> (x-y=w911:u16)
        n518 = Number To Boolean Array(number=w900) -> (Boolean array=w901:bool[])
        n519 = Or Array Elements(Boolean array=w901) -> (logical OR=w899:bool)
        n520 = Boolean To (0,1)(Boolean="+ phase (APD 1 Gate)") -> (0, 1=w909:i16)
        n521 = Boolean To (0,1)(Boolean=w899) -> (0, 1=w906:i16)
        n522 = Multiply(x=w909, y="Phase count adjustment (APD 1 Gate)") -> (x*y=w907:i16)
        n523 = To Unsigned Byte Integer(number=w906) -> (unsigned 8bit integer=w903:u8)
        n524 = Add(x=w911, y=w907) -> (x+y=w912:u16)
        n525 = feedback #40(i16 0) -> (w914:i16)
        n526 = Subtract(x=w914, y=w907) -> (x-y=w913:i16)
        "APD 1 Gate Relative Phase" <- w913
        n527 = feedback-in #40(w913) -> ()
        n528 = feedback #41(u8 0) -> (w904:u8)
        n529 = Add(x=w903, y=w904) -> (x+y=w902:u8)
        "APD 1 Gate Late Counter" <- w902
        n530 = feedback-in #41(w902) -> ()
        n531 = case shown="2" "APD Gate Operating Mode" {
          tunnel: [TRUE FALSE w933] -> w916
          tunnel: w919 -> [_ _ w930]
          frame 0, Default {
          }
          frame 1 {
          }
          frame 2 {
            n532 = Not(x=w930) -> (.not. x?=w932:bool)
            n533 = Select(t=w932, s="Invert APD Gate", f=w930) -> (s? t:f=w933:bool)
          }
        }
      }
    }
  }
  n534 = while "Control APD data integration - stream to host" {
    shift-right: [w937] -> _
    shift-left: w6 -> [w942]
    stop <- FALSE stop-if-true
    n535 = flat-sequence {
      tunnel: w942 -> [w944]
      tunnel: [w945] -> w940
      tunnel: [w944] -> w938
      tunnel: [w955] -> w941
      tunnel: w940 -> [w955]
      tunnel: [w954] -> w939
      tunnel: w938 -> [w954]
      tunnel: [w953] -> w936
      tunnel: [w952] -> w935
      tunnel: [w946] -> w934
      tunnel: [w997] -> w937
      tunnel: w941 -> [w1007]
      tunnel: w939 -> [w1004]
      tunnel: w936 -> [w990]
      tunnel: w935 -> [w989]
      tunnel: w934 -> [w977]
      frame #0 {
        n536 = call "Loop Timer6"("Count(Ticks)"=w944) -> ("Tick Count(Ticks)"=w945:u32)
      }
      frame #1 {
        n537 = flat-sequence {
          tunnel: [w957] -> w951
          tunnel: w951 -> [w960]
          tunnel: [w964] -> w950
          tunnel: [w963] -> w949
          tunnel: [w960] -> w948
          tunnel: [w959] -> w947
          tunnel: [w971] -> w952
          tunnel: [w972] -> w953
          tunnel: w950 -> [w972]
          tunnel: w949 -> [w971]
          tunnel: w948 -> [w970]
          tunnel: w947 -> [w969]
          tunnel: [w969] -> w946
          frame #0 {
            # "use separate variable so each APD won't\nhave to wait to read"
            n538 = feedback #42(FALSE) -> (w956:bool)
            "APD1 out state" <- w956
            "APD2 out state" <- w956
            "APD3 out state" <- w956
            n539 = Not(x=w956) -> (.not. x?=w957:bool)
            n540 = feedback-in #42(w957) -> ()
          }
          frame #1 {
            n541 = local read "APD 3 Counts 1"() -> (w962:u32)
            n542 = local read "APD 3 Counts 0"() -> (w961:u32)
            n543 = local read "APD 1 Counts 1"() -> (w968:u32)
            n544 = local read "APD 1 Counts 0"() -> (w967:u32)
            n545 = local read "APD 2 Counts 1"() -> (w966:u32)
            n546 = local read "APD 2 Counts 0"() -> (w965:u32)
            n547 = Select(t=w962, s=w960, f=w961) -> (s? t:f=w959:u32)
            n548 = Select(t=w968, s=w960, f=w967) -> (s? t:f=w964:u32)
            n549 = Select(t=w966, s=w960, f=w965) -> (s? t:f=w963:u32)
          }
          frame #2 {
            n550 = case shown="False" w970 {
              frame False {
                w973 = u32 0 ("APD 1 Counts 0")
                n551 = local write "APD 1 Counts 0"(w973) -> ()
                n552 = local write "APD 2 Counts 0"(w973) -> ()
                n553 = local write "APD 3 Counts 0"(w973) -> ()
              }
              frame True {
                w974 = u32 0 ("APD 1 Counts 1")
                n554 = local write "APD 1 Counts 1"(w974) -> ()
                n555 = local write "APD 2 Counts 1"(w974) -> ()
                n556 = local write "APD 3 Counts 1"(w974) -> ()
              }
            }
          }
        }
      }
      frame #2 {
        n557 = feedback-in #43(w1007) -> ()
        n558 = feedback #43(w1007) -> (w1006:u32)
        n559 = Subtract(x=w1007, y=w1006) -> (x-y=w1005:u32)
        n560 = Subtract(x=w1005, y=w1004) -> (x-y=w982:u32)
        n561 = case shown="True" "APD to FIFO" {
          tunnel: w990 -> [_ w1012]
          tunnel: w989 -> [_ w1010]
          tunnel: w977 -> [_ w1008]
          frame False {
          }
          frame True {
            n562 = flat-sequence {
              tunnel: 0 ("Timeout") -> [w1014]
              tunnel: w1012 -> [w1015]
              tunnel: [w1014] -> w1011
              tunnel: w1011 -> [w1016]
              tunnel: w1010 -> [w1017]
              tunnel: [w1016] -> w1009
              tunnel: w1009 -> [w1019]
              tunnel: w1008 -> [w1018]
              frame #0 {
                n563 = xnode ("FIFO Write")("Element"=w1015, "Timeout"=w1014) -> ()  [unwired: 1 in, 2 out]
              }
              frame #1 {
                n564 = xnode ("FIFO Write")("Element"=w1017, "Timeout"=w1016) -> ()  [unwired: 1 in, 2 out]
              }
              frame #2 {
                n565 = xnode ("FIFO Write")("Element"=w1018, "Timeout"=w1019) -> ()  [unwired: 1 in, 2 out]
              }
            }
          }
        }
        n566 = Subtract(x="APD Acq Rate Count", y=w982) -> (x-y=w998:u32)
        n567 = Number To Boolean Array(number=w982) -> (Boolean array=w983:bool[])
        n568 = Or Array Elements(Boolean array=w983) -> (logical OR=w981:bool)
        n569 = Boolean To (0,1)(Boolean=w981) -> (0, 1=w988:i16)
        n570 = To Unsigned Byte Integer(number=w988) -> (unsigned 8bit integer=w985:u8)
        n571 = feedback #44(u8 0) -> (w986:u8)
        n572 = Add(x=w985, y=w986) -> (x+y=w984:u8)
        "APD Acq Late Counter" <- w984
        n573 = feedback-in #44(w984) -> ()
        n574 = Boolean To (0,1)(Boolean="+ phase (APD Acq)") -> (0, 1=w994:i16)
        n575 = Multiply(x=w994, y="Phase Count Adjustment (APD Acq)") -> (x*y=w991:i16)
        n576 = Add(x=w998, y=w991) -> (x+y=w997:u32)
        n577 = feedback #45(i16 0) -> (w996:i16)
        n578 = Subtract(x=w996, y=w991) -> (x-y=w993:i16)
        "APD Acq Relative Phase" <- w993
        n579 = feedback-in #45(w993) -> ()
        n580 = To Word Integer(number=w990) -> (16bit integer=w999:i16)
        n581 = To Word Integer(number=w977) -> (16bit integer=w978:i16)
        n582 = To Word Integer(number=w989) -> (16bit integer=w1000:i16)
        n583 = Multiply(x="APD AO scale factor", y=w1000) -> (x*y=w979:i16)
        n584 = Multiply(x="APD AO scale factor", y=w978) -> (x*y=w975:i16)
        n585 = Multiply(x="APD AO scale factor", y=w999) -> (x*y=w980:i16)
        n586 = xnode "FPGA I/O Node"("Connector0/AO5"=w980, "Connector0/AO7"=w979, "Connector0/AO6"=w975) -> ()  [unwired: 3 in, 3 out]
      }
    }
  }
  n587 = while "DAQ AI set 1" {
    shift-right: [w1020] -> _
    shift-left: w1 -> [w1025]
    stop <- FALSE stop-if-true
    n588 = flat-sequence {
      tunnel: w1025 -> [w1035]
      tunnel: [w1036] -> w1023
      tunnel: [w1035] -> w1022
      tunnel: [w1046] -> w1033
      tunnel: [w1045] -> w1032
      tunnel: [w1044] -> w1031
      tunnel: [w1043] -> w1030
      tunnel: [w1042] -> w1029
      tunnel: [w1041] -> w1028
      tunnel: [w1040] -> w1027
      tunnel: [w1039] -> w1026
      tunnel: [w1038] -> w1024
      tunnel: w1023 -> [w1038]
      tunnel: w1022 -> [w1037]
      tunnel: [w1037] -> w1021
      tunnel: [w1075] -> w1020
      tunnel: w1033 -> [w1102]
      tunnel: w1032 -> [w1067]
      tunnel: w1031 -> [w1068]
      tunnel: w1030 -> [w1101]
      tunnel: w1029 -> [w1091]
      tunnel: w1028 -> [w1090]
      tunnel: w1027 -> [w1089]
      tunnel: w1026 -> [w1088]
      tunnel: w1024 -> [w1085]
      tunnel: w1021 -> [w1082]
      frame #0 {
        n589 = call "Loop Timer3"("Count(Ticks)"=w1035) -> ("Tick Count(Ticks)"=w1036:u16)
      }
      frame #1 {
        n590 = xnode "FPGA I/O Node"("Connector1/DIO31"=TRUE ("Connector1/DIO33")) -> ("Connector0/AI0"=w1046:i16, "Connector0/AI1"=w1045:i16, "Connector0/AI2"=w1044:i16, "Connector0/AI3"=w1043:i16, "Connector0/AI4"=w1042:i16, "Connector0/AI5"=w1041:i16, "Connector0/AI6"=w1040:i16, "Connector0/AI7"=w1039:i16)  [unwired: 9 in, 9 out]
      }
      frame #2 {
        w1071 = FALSE ("AI to FIFO")
        # "Adjust phase after data acquired if button pressed"
        n591 = feedback #46(i16 1) -> (w1094:i16)
        n592 = Increment(x=w1094) -> (x+1=w1100:i16)
        n593 = Scale By Power Of 2(n="AI1 X Scale", x=w1067) -> (x*2^n=w1065:i16)
        n594 = Greater?(x=w1100, y="N of AI1 Int Acq Sets") -> (0:w1097:bool)
        n595 = Select(t=i16 1, s=w1097, f=w1100) -> (s? t:f=w1099:i16)
        n596 = feedback-in #46(w1099) -> ()
        n597 = Divide(x=w1065, y=w1068) -> (x/y=w1064:fxp<+/-,16,1>)
        n598 = feedback #47(w1071) -> (w1069:bool)
        n599 = feedback #48(w1071) -> (w1087:bool)
        n600 = case shown="2" w1094 {
          tunnel: w1068 -> [w1125 w1132 _]
          tunnel: ["Set 1" "Set 2" "Set 3"] -> w1092
          tunnel: ["AI to FIFO" w1134 w1139] -> w1086
          tunnel: w1087 -> [_ w1134 w1139]
          tunnel: ["Trap Pos to FIFO" w1133 w1138] -> w1070
          tunnel: w1069 -> [_ w1133 w1138]
          tunnel: w1064 -> [w1124 w1131 _]
          tunnel: [w1123 w1129 FALSE] -> w1051
          tunnel: [w1122 w1130 u64 0 ("BD1 Frequency Out 2")] -> w1050
          frame 1, Default {
            n601 = local read "BD1 Frequency Out 1"() -> (w1122:u64)
            n602 = Compound Arithmetic op=AND("Trap Pos to FIFO", "Set 1", "AI to FIFO") -> (w1123:bool)
            "AI2 Y Sum Set 1" <- w1125
            "AI1 X Set 1" <- w1124
          }
          frame 2 {
            n603 = local read "BD1 Frequency Out 2"() -> (w1130:u64)
            n604 = Compound Arithmetic op=AND(w1133, "Set 2", w1134) -> (w1129:bool)
            "AI2 Y Sum Set 2" <- w1132
            "AI1 X Set 2" <- w1131
          }
          frame 3 {
          }
        }
        n605 = And(x=w1092, y=w1086) -> (x .and. y?=w1093:bool)
        n606 = case shown="True" w1093 {
          tunnel: w1102 -> [_ w1153]
          tunnel: w1067 -> [_ w1152]
          tunnel: w1068 -> [_ w1151]
          tunnel: w1101 -> [_ w1150]
          tunnel: w1091 -> [_ w1149]
          tunnel: w1090 -> [_ w1148]
          tunnel: w1089 -> [_ w1147]
          tunnel: w1088 -> [_ w1146]
          tunnel: 0 ("DMA buffer timeout") -> [_ w1155]
          frame False {
          }
          frame True {
            n607 = Build Array(w1153, w1152, w1151, w1150, w1149, w1148, w1147, w1146) -> (w1154:i16[])
            n608 = for {
              tunnel: w1154 -> [w1157] mode=indexing
              tunnel: w1155 -> [w1158]
              tunnel: [w1156] -> w1144 mode=indexing
              n609 = xnode ("FIFO Write")("Element"=w1157, "Timeout"=w1158) -> ("Timed Out?"=w1156:bool)  [unwired: 1 in, 1 out]
            }
            n610 = Or Array Elements(Boolean array=w1144) -> (logical OR=w1141:bool)
            n611 = Boolean To (0,1)(Boolean=w1141) -> (0, 1=w1143:i16)
            n612 = feedback #49(u16 0) -> (w1142:u16)
            n613 = Add(x=w1143, y=w1142) -> (x+y=w1140:u16)
            "Trap AI FIFO Timeout" <- w1140
            n614 = feedback-in #49(w1140) -> ()
          }
        }
        n615 = feedback-in #47(w1070) -> ()
        n616 = feedback-in #48(w1086) -> ()
        n617 = case shown="True" w1051 {
          tunnel: w1050 -> [_ w1108]
          tunnel: [u8 0 w1105] -> w1049
          frame False {
          }
          frame True {
            n618 = Split Number(x=w1108) -> (hi(x)=w1109:u32, lo(x)=w1110:u32)
            n619 = Split Number(x=w1109) -> (lo(x)=w1111:u16)  [unwired: 1 out]
            n620 = Split Number(x=w1110) -> (hi(x)=w1112:u16, lo(x)=w1113:u16)
            n621 = Build Array "BD 1 nu Stack"(w1111, w1112, w1113) -> (w1107:u16[])
            n622 = for {
              tunnel: w1107 -> [w1120] mode=indexing
              shift-right: [w1116] -> w1105
              shift-left: u8 0 -> [w1117]
              n623 = xnode ("FIFO Method Node")("Element"=w1120, "Timeout"="Trap FIFO Set Timeout") -> ("Timed Out?"=w1119:bool)  [unwired: 1 in, 1 out]
              n624 = Boolean To (0,1)(Boolean=w1119) -> (0, 1=w1118:i16)
              n625 = To Unsigned Byte Integer(number=w1118) -> (unsigned 8bit integer=w1115:u8)
              n626 = Add(x=w1115, y=w1117) -> (x+y=w1116:u8)
            }
          }
        }
        n627 = To Unsigned Word Integer(number=w1049) -> (unsigned 16bit integer=w1048:u16)
        n628 = feedback #50(u16 0) -> (w1062:u16)
        n629 = Add(x=w1048, y=w1062) -> (x+y=w1061:u16)
        "Trap Pos FIFO Timeout" <- w1061
        n630 = feedback-in #50(w1061) -> ()
        n631 = feedback-in #51(w1085) -> ()
        n632 = feedback #51(w1085) -> (w1084:u16)
        n633 = Subtract(x=w1085, y=w1084) -> (x-y=w1083:u16)
        n634 = xnode "FPGA I/O Node"("Connector1/DIO31"=FALSE ("Connector1/DIO34")) -> ()  [unwired: 1 in, 1 out]
        n635 = Subtract(x=w1083, y=w1082) -> (x-y=w1053:u16)
        n636 = Boolean To (0,1)(Boolean="+ phase") -> (0, 1=w1078:i16)
        n637 = Multiply(x=w1078, y="Phase count adjustment") -> (x*y=w1072:i16)
        n638 = Subtract(x="ai count", y=w1053) -> (x-y=w1076:u16)
        n639 = Number To Boolean Array(number=w1053) -> (Boolean array=w1054:bool[])
        n640 = feedback #52(i16 0) -> (w1074:i16)
        n641 = Add(x=w1076, y=w1072) -> (x+y=w1075:u16)
        n642 = Subtract(x=w1074, y=w1072) -> (x-y=w1073:i16)
        "Relative phase" <- w1073
        n643 = feedback-in #52(w1073) -> ()
        n644 = Or Array Elements(Boolean array=w1054) -> (logical OR=w1052:bool)
        n645 = Boolean To (0,1)(Boolean=w1052) -> (0, 1=w1059:i16)
        n646 = To Unsigned Byte Integer(number=w1059) -> (unsigned 8bit integer=w1056:u8)
        n647 = feedback #53(u8 0) -> (w1057:u8)
        n648 = Add(x=w1056, y=w1057) -> (x+y=w1055:u8)
        "AI Late Counter" <- w1055
        n649 = feedback-in #53(w1055) -> ()
      }
    }
  }
  n650 = node-c288(w7) -> ()
  n651 = while "APD 3 Counter" {
    tunnel: w1 -> [_]
    stop <- FALSE stop-if-true
    n652 = flat-sequence {
      frame #0 {
        n653 = xnode "FPGA I/O Method Node"("FPGA I/O In"=refnum<k21> "Connector0/DIO2" ("APD 2 DO"), "Timeout"=-1) -> ()  [unwired: 2 out]
      }
      frame #1 {
        n654 = local read "APD3 out state"() -> (w1162:bool)
        n655 = case shown="False" w1162 {
          frame False {
            n656 = local read "APD 3 Counts 0"() -> (w1164:u32)
            n657 = Increment(x=w1164) -> (x+1=→"APD 3 Counts 0":u32)
          }
          frame True {
            n658 = local read "APD 3 Counts 1"() -> (w1166:u32)
            n659 = Increment(x=w1166) -> (x+1=→"APD 3 Counts 1":u32)
          }
        }
      }
    }
  }
  n660 = while "APD 3 Gating" {
    shift-right: [w1170] -> _
    shift-left: w1 -> [w1175]
    shift-right: [w1169] -> _
    shift-left: w5 -> [w1167]
    stop <- FALSE stop-if-true
    n661 = flat-sequence {
      tunnel: w1175 -> [w1178]
      tunnel: [w1179] -> w1173
      tunnel: [w1178] -> w1171
      tunnel: [w1177] -> w1168
      tunnel: w1167 -> [w1177]
      tunnel: [w1182] -> w1174
      tunnel: w1173 -> [w1182]
      tunnel: [w1181] -> w1172
      tunnel: w1171 -> [w1181]
      tunnel: w1168 -> [w1180]
      tunnel: [w1199] -> w1170
      tunnel: w1174 -> [w1211]
      tunnel: w1172 -> [w1208]
      tunnel: [w1203] -> w1169
      frame #0 {
        n662 = call "Loop Timer15"("Count(Ticks)"=w1178) -> ("Tick Count(Ticks)"=w1179:u16)
      }
      frame #1 {
        # "Signal is then sent through \na transistor before APD"
        n663 = xnode "FPGA I/O Node"("Connector0/DIO9"=w1180) -> ()  [unwired: 1 in, 1 out]
      }
      frame #2 {
        n664 = local read "APD Gate OFF Count"() -> (w1184:u16)
        n665 = local read "APD Gate ON Count"() -> (w1185:u16)
        n666 = feedback #54(TRUE) -> (w1205:bool)
        n667 = feedback-in #55(w1211) -> ()
        n668 = feedback #55(w1211) -> (w1210:u16)
        n669 = Not(x=w1205) -> (.not. x?=w1202:bool)
        n670 = feedback-in #54(w1202) -> ()
        n671 = Subtract(x=w1211, y=w1210) -> (x-y=w1209:u16)
        n672 = Select(t=w1185, s=w1202, f=w1184) -> (s? t:f=w1207:u16)
        n673 = Subtract(x=w1209, y=w1208) -> (x-y=w1187:u16)
        n674 = Subtract(x=w1207, y=w1187) -> (x-y=w1198:u16)
        n675 = Number To Boolean Array(number=w1187) -> (Boolean array=w1188:bool[])
        n676 = Or Array Elements(Boolean array=w1188) -> (logical OR=w1186:bool)
        n677 = Boolean To (0,1)(Boolean=w1186) -> (0, 1=w1193:i16)
        n678 = Boolean To (0,1)(Boolean="+ phase (APD 3 Gate)") -> (0, 1=w1196:i16)
        n679 = To Unsigned Byte Integer(number=w1193) -> (unsigned 8bit integer=w1190:u8)
        n680 = Multiply(x=w1196, y="Phase count adjustment (APD 3 Gate)") -> (x*y=w1194:i16)
        n681 = feedback #56(u8 0) -> (w1191:u8)
        n682 = Add(x=w1190, y=w1191) -> (x+y=w1189:u8)
        "APD 3 Gate Late Counter" <- w1189
        n683 = feedback-in #56(w1189) -> ()
        n684 = Add(x=w1198, y=w1194) -> (x+y=w1199:u16)
        n685 = feedback #57(i16 0) -> (w1201:i16)
        n686 = Subtract(x=w1201, y=w1194) -> (x-y=w1200:i16)
        "APD 3 Gate Relative Phase" <- w1200
        n687 = feedback-in #57(w1200) -> ()
        n688 = local read "APD Gate Operating Mode"() -> (w1183:u8)
        n689 = case shown="2" w1183 {
          tunnel: [TRUE FALSE w1217] -> w1203
          tunnel: w1205 -> [_ _ w1215]
          frame 0, Default {
          }
          frame 1 {
          }
          frame 2 {
            n690 = local read "Invert APD Gate"() -> (w1214:bool)
            n691 = Not(x=w1215) -> (.not. x?=w1216:bool)
            n692 = Select(t=w1216, s=w1214, f=w1215) -> (s? t:f=w1217:bool)
          }
        }
      }
    }
  }
  n693 = while "633 nm red  fluorescent laser interlacing (DO to IA 633 nm AOM ME amp)." {
    shift-right: [w1221] -> _
    shift-left: w1 -> [w1226]
    shift-right: [w1220] -> _
    shift-left: w2 -> [w1218]
    stop <- FALSE stop-if-true
    n694 = flat-sequence {
      tunnel: w1226 -> [w1229]
      tunnel: [w1230] -> w1224
      tunnel: [w1229] -> w1222
      tunnel: [w1228] -> w1219
      tunnel: w1218 -> [w1228]
      tunnel: [w1233] -> w1225
      tunnel: w1224 -> [w1233]
      tunnel: [w1232] -> w1223
      tunnel: w1222 -> [w1232]
      tunnel: w1219 -> [w1231]
      tunnel: [w1242] -> w1221
      tunnel: w1225 -> [w1262]
      tunnel: w1223 -> [w1259]
      tunnel: [w1251] -> w1220
      frame #0 {
        n695 = call "Loop Timer11"("Count(Ticks)"=w1229) -> ("Tick Count(Ticks)"=w1230:u16)
      }
      frame #1 {
        # "Then to PRL 440 amp"
        n696 = xnode "FPGA I/O Node"("Connector1/DIO32"=w1231) -> ()  [unwired: 1 in, 1 out]
      }
      frame #2 {
        n697 = feedback-in #58(w1262) -> ()
        n698 = feedback #58(w1262) -> (w1261:u16)
        n699 = Subtract(x=w1262, y=w1261) -> (x-y=w1260:u16)
        n700 = Subtract(x=w1260, y=w1259) -> (x-y=w1235:u16)
        n701 = Number To Boolean Array(number=w1235) -> (Boolean array=w1236:bool[])
        n702 = Or Array Elements(Boolean array=w1236) -> (logical OR=w1234:bool)
        n703 = Boolean To (0,1)(Boolean="+ phase (RI)") -> (0, 1=w1247:i16)
        n704 = Multiply(x=w1247, y="Phase count adjustment (RI)") -> (x*y=w1244:i16)
        n705 = Boolean To (0,1)(Boolean=w1234) -> (0, 1=w1241:i16)
        n706 = To Unsigned Byte Integer(number=w1241) -> (unsigned 8bit integer=w1238:u8)
        n707 = feedback #59(i16 0) -> (w1245:i16)
        n708 = feedback #60(u8 0) -> (w1239:u8)
        n709 = Add(x=w1238, y=w1239) -> (x+y=w1237:u8)
        "RI Late Counter" <- w1237
        n710 = feedback-in #60(w1237) -> ()
        n711 = Subtract(x=w1245, y=w1244) -> (x-y=w1243:i16)
        "RI Relative phase" <- w1243
        n712 = feedback-in #59(w1243) -> ()
        n713 = feedback #61(TRUE) -> (w1254:bool)
        n714 = case shown="2" "Red Laser Operating Mode" {
          tunnel: [TRUE FALSE w1268] -> w1251
          tunnel: w1254 -> [_ _ w1265]
          frame 0, Default {
          }
          frame 1 {
          }
          frame 2 {
            n715 = Not(x=w1265) -> (.not. x?=w1267:bool)
            n716 = Select(t=w1267, s="Invert RI", f=w1265) -> (s? t:f=w1268:bool)
          }
        }
        n717 = Not(x=w1254) -> (.not. x?=w1250:bool)
        n718 = Select(t="Red interlace ON count", s=w1250, f="Red interlace OFF count") -> (s? t:f=w1256:u16)
        n719 = Subtract(x=w1256, y=w1235) -> (x-y=w1248:u16)
        n720 = Add(x=w1248, y=w1244) -> (x+y=w1242:u16)
        n721 = feedback-in #61(w1250) -> ()
      }
    }
  }
  n722 = while "473 nm blue  fluorescent laser interlacing (DO to blue laser digital control input)." {
    shift-right: [w1272] -> _
    shift-left: w1 -> [w1277]
    shift-right: [w1271] -> _
    shift-left: w2 -> [w1269]
    stop <- FALSE stop-if-true
    n723 = flat-sequence {
      tunnel: w1277 -> [w1280]
      tunnel: [w1281] -> w1275
      tunnel: [w1280] -> w1273
      tunnel: [w1279] -> w1270
      tunnel: w1269 -> [w1279]
      tunnel: [w1284] -> w1276
      tunnel: w1275 -> [w1284]
      tunnel: [w1283] -> w1274
      tunnel: w1273 -> [w1283]
      tunnel: w1270 -> [w1282]
      tunnel: [w1293] -> w1272
      tunnel: w1276 -> [w1313]
      tunnel: w1274 -> [w1310]
      tunnel: [w1302] -> w1271
      frame #0 {
        n724 = call "Loop Timer14"("Count(Ticks)"=w1280) -> ("Tick Count(Ticks)"=w1281:u16)
      }
      frame #1 {
        n725 = xnode "FPGA I/O Node"("Connector1/DIO28"=w1282) -> ()  [unwired: 1 in, 1 out]
      }
      frame #2 {
        n726 = feedback-in #62(w1313) -> ()
        n727 = feedback #62(w1313) -> (w1312:u16)
        n728 = Subtract(x=w1313, y=w1312) -> (x-y=w1311:u16)
        n729 = Subtract(x=w1311, y=w1310) -> (x-y=w1286:u16)
        n730 = Number To Boolean Array(number=w1286) -> (Boolean array=w1287:bool[])
        n731 = Or Array Elements(Boolean array=w1287) -> (logical OR=w1285:bool)
        n732 = Boolean To (0,1)(Boolean="+ phase (BI D)") -> (0, 1=w1298:i16)
        n733 = Multiply(x=w1298, y="Phase count adjustment (BI D)") -> (x*y=w1295:i16)
        n734 = Boolean To (0,1)(Boolean=w1285) -> (0, 1=w1292:i16)
        n735 = To Unsigned Byte Integer(number=w1292) -> (unsigned 8bit integer=w1289:u8)
        n736 = feedback #63(i16 0) -> (w1296:i16)
        n737 = feedback #64(u8 0) -> (w1290:u8)
        n738 = Add(x=w1289, y=w1290) -> (x+y=w1288:u8)
        "Blue Late Counter (D)" <- w1288
        n739 = feedback-in #64(w1288) -> ()
        n740 = Subtract(x=w1296, y=w1295) -> (x-y=w1294:i16)
        "BI Relative phase (D)" <- w1294
        n741 = feedback-in #63(w1294) -> ()
        n742 = feedback #65(TRUE) -> (w1305:bool)
        n743 = case shown="2" "Blue Laser Operating Mode (D)" {
          tunnel: [TRUE FALSE w1319] -> w1302
          tunnel: w1305 -> [_ _ w1316]
          frame 0, Default {
          }
          frame 1 {
          }
          frame 2 {
            n744 = Not(x=w1316) -> (.not. x?=w1318:bool)
            n745 = Select(t=w1318, s="Invert BI (D)", f=w1316) -> (s? t:f=w1319:bool)
          }
        }
        n746 = Not(x=w1305) -> (.not. x?=w1301:bool)
        n747 = Select(t="Blue interlace ON count (D)", s=w1301, f="Blue interlace OFF count (D)") -> (s? t:f=w1307:u16)
        n748 = Subtract(x=w1307, y=w1286) -> (x-y=w1299:u16)
        n749 = Add(x=w1299, y=w1295) -> (x+y=w1293:u16)
        n750 = feedback-in #65(w1301) -> ()
      }
    }
  }
  n751 = while "Blue fluorescent laser interlacing (AO control direct to laser)." {
    shift-right: [w1325] -> _
    shift-left: w1 -> [w1328]
    shift-right: [w1322] -> _
    shift-left: i16 0 -> [w1320]
    stop <- FALSE stop-if-true
    n752 = flat-sequence {
      tunnel: w1328 -> [w1331]
      tunnel: [w1332] -> w1327
      tunnel: [w1331] -> w1326
      tunnel: [w1330] -> w1321
      tunnel: w1320 -> [w1330]
      tunnel: [w1335] -> w1324
      tunnel: w1327 -> [w1335]
      tunnel: [w1334] -> w1323
      tunnel: w1326 -> [w1334]
      tunnel: w1321 -> [w1333]
      tunnel: [w1345] -> w1325
      tunnel: [w1361] -> w1322
      tunnel: w1324 -> [w1373]
      tunnel: w1323 -> [w1370]
      frame #0 {
        n753 = call "Loop Timer13"("Count(Ticks)"=w1331) -> ("Tick Count(Ticks)"=w1332:u16)
      }
      frame #1 {
        n754 = xnode "FPGA I/O Node"("Connector0/AO3"=w1333) -> ()  [unwired: 1 in, 1 out]
      }
      frame #2 {
        n755 = Subtract(x="Blue OFF count (AO)", y="Blue current ON count adj (AO)") -> (x-y=w1354:u16)
        n756 = feedback-in #66(w1373) -> ()
        n757 = feedback #66(w1373) -> (w1372:u16)
        n758 = Add(x="Blue current ON count adj (AO)", y="Blue ON count (AO)") -> (x+y=w1355:u16)
        n759 = Subtract(x=w1373, y=w1372) -> (x-y=w1371:u16)
        n760 = Subtract(x=w1371, y=w1370) -> (x-y=w1338:u16)
        n761 = Number To Boolean Array(number=w1338) -> (Boolean array=w1339:bool[])
        n762 = Boolean To (0,1)(Boolean="+ phase (BI AO)") -> (0, 1=w1351:i16)
        n763 = Or Array Elements(Boolean array=w1339) -> (logical OR=w1337:bool)
        n764 = Boolean To (0,1)(Boolean=w1337) -> (0, 1=w1344:i16)
        n765 = Multiply(x=w1351, y="Phase count adjustment (BI AO)") -> (x*y=w1347:i16)
        n766 = To Unsigned Byte Integer(number=w1344) -> (unsigned 8bit integer=w1340:u8)
        n767 = feedback #67(u8 0) -> (w1342:u8)
        n768 = Add(x=w1340, y=w1342) -> (x+y=w1341:u8)
        "BI Late Counter (AO)" <- w1341
        n769 = feedback-in #67(w1341) -> ()
        n770 = feedback #68(i16 0) -> (w1348:i16)
        n771 = Subtract(x=w1348, y=w1347) -> (x-y=w1346:i16)
        "BI Relative phase (AO)" <- w1346
        n772 = feedback-in #68(w1346) -> ()
        n773 = feedback #69(TRUE) -> (w1365:bool)
        n774 = case shown="2" "BI Operating Mode (AO)" {
          tunnel: [TRUE FALSE w1389] -> w1356
          tunnel: w1365 -> [_ _ w1386]
          frame 0, Default {
          }
          frame 1 {
          }
          frame 2 {
            n775 = Not(x=w1386) -> (.not. x?=w1388:bool)
            n776 = Select(t=w1388, s="Invert BI (AO)", f=w1386) -> (s? t:f=w1389:bool)
          }
        }
        n777 = And(x=w1356, y="Blue FB On/Off") -> (x .and. y?=w1357:bool)
        n778 = case shown="True" w1357 {
          tunnel: "BI Current Out" -> [w1374 _]
          tunnel: [w1374 w1376] -> w1360
          frame False {
          }
          frame True {
            n779 = local read "Blue Intensity"() -> (w1375:i16)
            n780 = Bundle("P5"="P5", "I5"="I5", "D5"="D5") -> (w1377:cluster{"P5":i16, "I5":i16, "D5":i16})  [unwired: 1 in]
            n781 = call "Slower PID.vi"("process variable"=w1375, "reset?"="Blue FB Reset", "setpoint"="Blue FB Setpoint", "PID gains (x 2^8)"=w1377, "output range"=cluster{"output high":i16, "output low":i16} {"output high"=32767, "output low"=0} ("Green FB output range")) -> ("output"=w1376:i16)  [unwired: 10 out]
          }
        }
        n782 = Not(x=w1365) -> (.not. x?=w1362:bool)
        n783 = Select(t=w1355, s=w1362, f=w1354) -> (s? t:f=w1367:u16)
        n784 = Subtract(x=w1367, y=w1338) -> (x-y=w1349:u16)
        n785 = Add(x=w1349, y=w1347) -> (x+y=w1345:u16)
        n786 = feedback-in #69(w1362) -> ()
        n787 = Boolean To (0,1)(Boolean=w1356) -> (0, 1=w1336:i16)
        n788 = Multiply(x=w1336, y=w1360) -> (x*y=w1361:i16)
      }
    }
  }
